vi "02 HEWH Heat Up Test SM1.vi"(0 "Equipment":T7={"COM Port"="COM3", "MW100"="MW100", "AG34970"="A-34972A", "Chamber"="WT500"}, 2 "Semiphore":T1, 5 "Degree Setting":dbl=58.0, 7 "Flow rate setting":dbl=3.0, 11 "Error In":errorcluster) -> (15 "Error Out":errorcluster)   [LabVIEW 2011]
uses:
  EquipReferences.ctl
  Heating Modes.ctl
  HEWH Tank Indicator.ctl
  PowerElements.ctl
  Use Modes.ctl
  TestedFlowratesScenarios.ctl
  GEA2/HEWH_Mode.ctl
  ValveBankPositions.ctl
  Intellifaucet/Intellfaucet Mode.ctl
  Global HEWH.vi
  <vilib>/Utility/file.llb/Write To Spreadsheet File (string).vi
  <vilib>/Analysis/NI_AALBase.lvlib
panel:
  in  "mS Between Serial Polls":u32=500
  out "Retries":i32
  out "Serial Read OK":bool
  out "GEA2":T1
  in  "Test Condition":T2=enum."Global, Tank"
  out "Chanel List":string
  out "Label Array":string[](array[string])
  out "Use Agilent?":bool
  out "Voltage":dbl=240.0
  out "T4":i32=10000
  out "COM Port":refnum<visa-resource-name>
  out "Serial Data In":string
  out "Error Serial":errorcluster
  in  "StopSerial":bool
  out "LAN IP Address":string="192.168.25.3"
  out "Computer Name":string
  in  "Mode Set?":bool
  out "Ver.":string
  out "HEATUP TEST STATUS":string
  in  "Stop":bool
  in  "Help":bool
  out "POWER":T3
  out "Tank Display":T4 {"TC6" format="%.2g"; "TIN" format="%.2g"; "TOUT" format="%.2g"; "Mean" format="%.2f"; "Std Dev" format="%.2f"; "TC5" format="%.2g"; "TC4" format="%.2g"; "TC3" format="%.2g"; "TC2" format="%.2g"; "TC1" format="%.2g"}
  in  "Function Tab":enum32{"Setup", "Test Status", "Charts"}(tab)
  out "MW100":refnum<visa-resource-name>
  out "FileName":path
  in  "Working File Directory":path=path "c:/data"
  out "T1":u32=250
  out "T2":u32=500
  out "T3":u32=500
  in  "Cold Water Available?":bool=TRUE
  out "Heating  Mode":T5=enum."Hybrid Heating"
  in  "DRM Mode":T6=3 items=["CRITICAL", "HIGH", "MEDIUM", "Normal"]
  in  "Save File Directory":path=path "c:/data"
  out "Data Array":string[][](array[string])
  out "GEA2 HyperData":bool=TRUE
  in  "Expansion Tank?":bool=TRUE
  in  "Com Err Limit":dbl=20.0
  in  "Status Tab":T8(tab)=enum."Feedback 6"
  out "errorset mode":errorcluster
  out "Init Complete":bool
  out "Mode":T9=enum."HighDemand"
  out "Set Point":u8=140
  out "Heat Source Indicator":bool
  in  "SkipStabilize":bool
  out "error stabilize":errorcluster
  out "Elapsed Time (secs)":dbl format="%.2f"
  in  "Stability Sample Delay(s)":dbl=120.0
  out "1.Delay Mins(30)":dbl
  in  "1.SkipDelay":bool
  out "Flowrate adj":dbl=3.0
  out "Error Out 1":errorcluster
  out "Downspout Flow Chart":dbl(graph)=3.8899999999999997
  out "Temp Band(+/- F)":dbl=50.0
  in  "Time Delay(30)":dbl=30.0
  out "Temp adj":dbl=3.0
  out "Downspout Temp":dbl(graph)=3.8899999999999997
  out "2.Bottom Source Indicator":bool
  out "2.TotWater":dbl
  in  "2. Initial Draw":dbl=10.75
  out "3.WaitTime(10min)":dbl
  out "error 3":errorcluster
  out "3.Heat Source Indicator":bool
  in  "Wait Time(600s)":dbl=600.0
  out "4.Delay Remaining (300s)":dbl
  in  "Delay(300s)":dbl=300.0
  in  "4.Skip Delay":bool
  out "Error 5":errorcluster
  out "Downspout Flow Chart":dbl(graph)=3.8899999999999997
  out "Downspout Flow":dbl=3.8899999999999997
  out "Total Gal Out":dbl
  out "5.Top Source Indicator":bool
  in  "Eheat Gal Limit":dbl=40.0
  in  "Flow Adjust Time (3s)":dbl=1.5
  in  "K(0.1)":dbl=0.1
  in  "Total Gal Limit":dbl=200.0
  out "6.Bottom Source Indicator":bool
  in  "Skip Waiting for Bottom Source to turn off.":bool
  out "7.Heat Source Indicator":bool
  out "Mean Tank Temp":dbl
  in  "Min Ave Temp Limit":dbl=120.0
  in  "8.Skip Waiting":bool
  out "Seconds to Completion":dbl
  in  "8.Delay(1800s)":dbl=1800.0
  out "LoggingStopped":bool=TRUE
  out "Error History":string[](array[string])
  out "Com History":string[](array[string])
  out "error datalogging":errorcluster={"status"=TRUE, "code"=-1073807346, "source"="VISA Read in Gather Test Data.vi"}
  out "St.Logging":bool
  out "Number of Records":i32
  out "Test Data":string[][](array[string])
  in  "Graph Tab":enum32{"Temperature", "Power", "Gallons"}(tab)
  out "Temps":T10(graph) caption="Waveform Chart"
  out "Ave Temp":dbl format="%0.2f"
  out "Watt Chart":T11(graph)
  out "Watts":dbl
  out "Gallons Chart":dbl(graph)
  out "Gallons":dbl
  out "Elapsed Time":dbl format="%<%H:%M:%S>t"
  in  "Stop Logging":bool
  out "Local?":bool
  # "Select the Modes for the test.  This will need to be\nset up on the water heater."
  # "Wait for stabilization.  Checks heat sources every second.  \nIf the heat sources are both off, the water heater is stabilized. \nFor StdElect. Looks at the heating element.  For other heating\nmodes, looks at the RS232 feedback on fans and compressor."
  # "\"1.\tAfter unit has been stable for 30+/-5 minutes, Open valve,\n and draw 10.75 +/- .25 gallons of water at a rate of 3+/-.25 gpm.\""
  # "First, Allow the water temp and flow to stabilize in the downspout,\nthen switch to the tank."
  # "\"2.\tIf lower heat source energizes (Hybrid Mode/eHeat Mode = FAN ON\nfollow by Compressor, Standard Electric Mode = Lower Element ON) \nbefore 10.75 gallons, then continue drawing water until Upper element \nengages as shown in step 5 (skip to step 5).\""
  # "\"3.\tIf lower heat source does not energize during 10.75 gallon draw, then wait a maximum of 10 minutes to see if lower heat source will energize.  If it does, then\nallow the water heater to recover to set point.\""
  # "\"4.\tAllow unit to sit 5 to 10 minutes in stabilized conditions, then:\""
  # "Change delay value to skip ahead."
  # "\"5.\tOpen valve and draw water at 3+/-.25 gpm until the Upper Element \nenergizes.  Water draw must stop within 5 seconds after Upper Element \nenergizes.  NOTE: when running the unit in e-Heat mode, (no upper \nelement) draw 40+/-0.25 gallons of water.\""
  # "\"6.\tIn Hybrid Mode: when the Upper Element stops and \nswitches to Lower Element, switch the unit to eHeat Mode.  \nThis will switch the lower heating source to Compressor.\""
  # "Since there may be a significant delay \nfor the compressor to turn on, also check \nto make sure that the mean tank temp\nis above some limit."
  # "7.\tAllow water heater to stabilize this second time. \n(Recover water temperature back to set point)."
  # "8.\tAllow unit to sit a minimum of 30 minutes in stabilized conditions, then;"
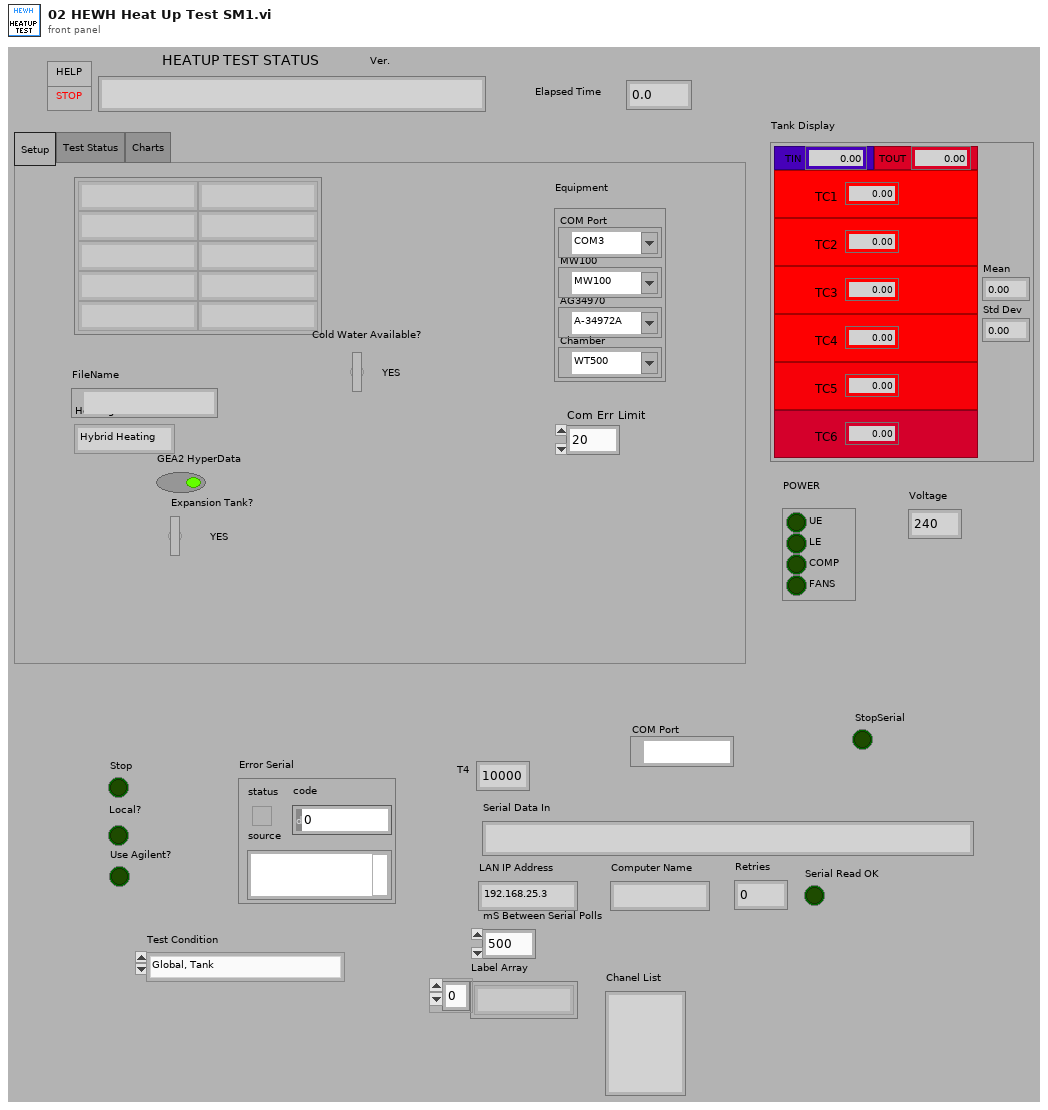
[diagram p1: front panel]
types:
  T1 = typedef "Semaphore RefNum" = refnum<k1>
  T2 = typedef "TestedFlowratesScenarios.ctl" = enum16{"DRK500,Station1", "DRK375,Lab", "SRK500,Station1,5GPM FR", "DRK375,STATION3,1/2\"HOSE", "DRK500,Station1,downspout", "DRK375,Station3,thruEcocute", "DRK375,Station3,purge", "Build2,2B,Purge", "Global, Purge", "Global, Tank"}
  T3 = typedef "PowerElements.ctl" = cluster{"UE":bool, "LE":bool, "COMP":bool, "FANS":bool}
  T4 = typedef "HEWH Tank Indicator.ctl" = cluster{"TC1-D":bool, "TC2-D":bool, "TC3-D":bool, "TC4-D":bool, "TC5-D":bool, "RTD_IN":bool, "RTDOUT":bool, "TC1":dbl, "TC2":dbl, "TC3":dbl, "TC4":dbl, "TC5":dbl, "TIN":dbl, "TOUT":dbl, "Std Dev":dbl, "Mean":dbl, "TC6-D":bool, "TC6":dbl}
  T5 = typedef "Heating Modes.ctl" = enum16{"Standard Electric", "Hybrid Heating", "E-Heat Mode"}
  T6 = typedef "Use Modes.ctl" = u16
  T7 = typedef "EquipReferences.ctl" = cluster{"COM Port":refnum<visa-resource-name>, "MW100":refnum<visa-resource-name>, "AG34970":refnum<visa-resource-name>, "Chamber":refnum<visa-resource-name>}
  T8 = enum32{"External Program Controls", "External Program Controls 2", "Program Controls", "Feedback", "Feedback 2", "Feedback 3", "Feedback 4", "Feedback 5", "Feedback 6", "Feedback 7", "Feedback 8", "Feedback 9", "Feedback 10"}
  T9 = typedef "HEWH_Mode.ctl" = enum16{"Hybrid", "StdElectric", "eHeat", "HighDemand", "Vacation"}
  T10 = cluster{"Tc Tree[0]":dbl, "Tc Tree[1]":dbl, "Tc Tree[2]":dbl, "Tc Tree[3]":dbl, "Tc Tree[4]":dbl, "Tc Tree[5]":dbl}[]
  T11 = cluster{"[0]":dbl, "[1]":dbl, "[2]":dbl, "[3]":dbl, "[4]":dbl, "[5]":dbl}[]
  T12 = typedef "Intellfaucet Mode.ctl" = enum16{"Adjust Temp", "Adjust Flow", "Start Flow", "Stop Flow"}
  T13 = typedef "ValveBankPositions.ctl" = enum16{"Heating", "Purge", "Resting", "Draw"}
  T14 = enum16{"Computation Start", "Computation stop", "Reset Computation", "Clear Computation"}
  T15 = typedef "FileVersionInformation.ctl" = cluster{"FileVersion":string, "ProductName":string, "InternalName":string, "CompanyName":string, "LegalCopyright":string, "FileDescription":string}
  T16 = enum16{"Computation Start", "Computation stop", "Reset Computation", "Clear Computation"}[]
  T17 = typedef "PowerData.ctl" = cluster{"Voltage":dbl, "Current":dbl, "Power":dbl, "WattHours":dbl}
  T18 = cluster{"Tc Tree[0]":dbl, "Tc Tree[1]":dbl, "Tc Tree[2]":dbl, "Tc Tree[3]":dbl, "Tc Tree[4]":dbl, "Tc Tree[5]":dbl}
  T19 = cluster{"[0]":dbl, "[1]":dbl, "[2]":dbl, "[3]":dbl, "[4]":dbl, "[5]":dbl}
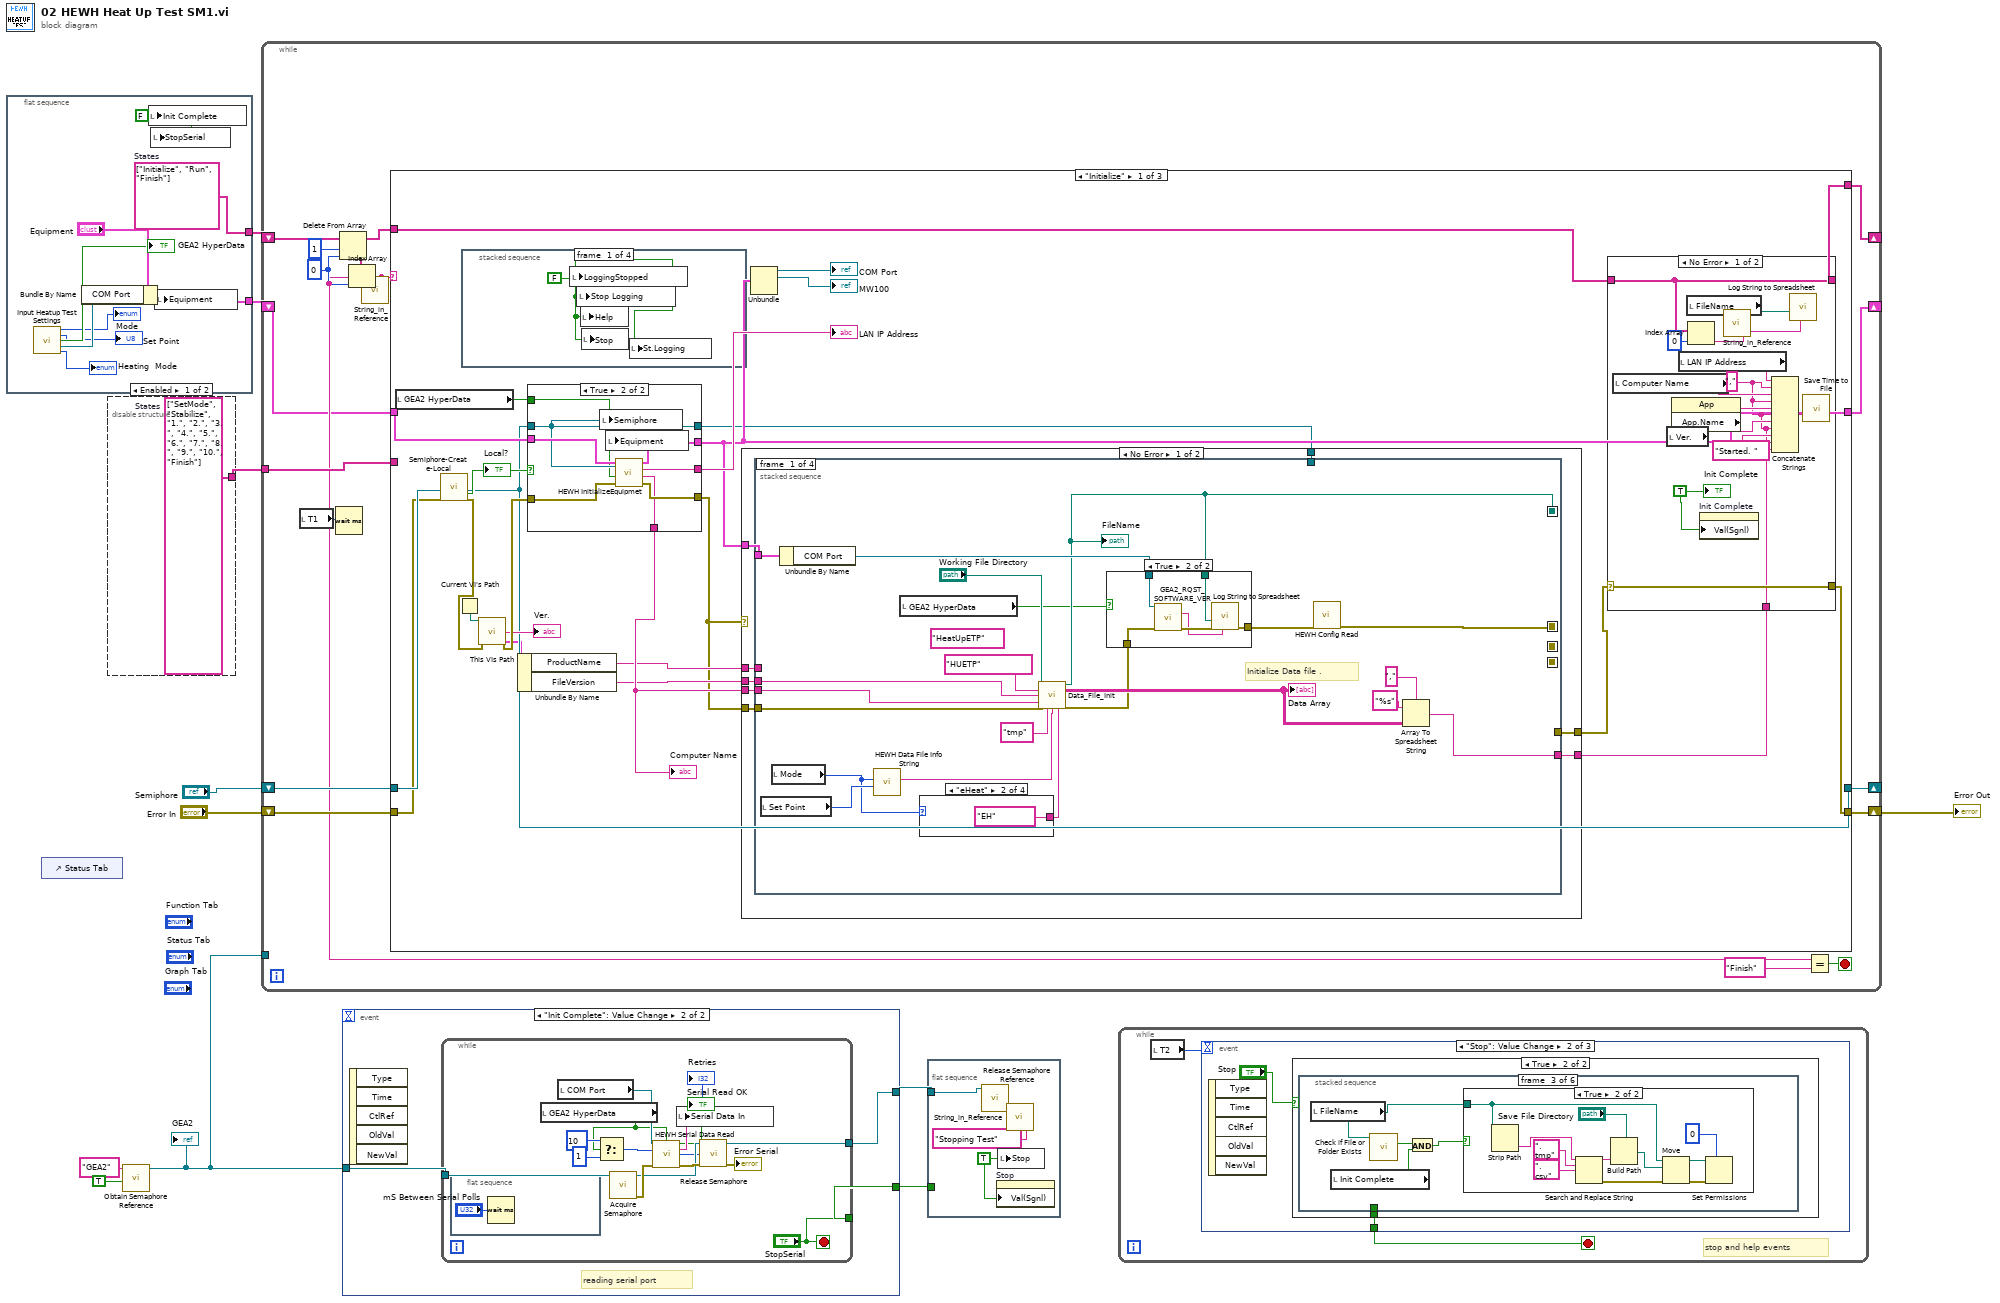
[diagram p0: block diagram]
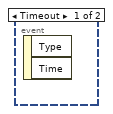
[diagram p2: hidden frame]
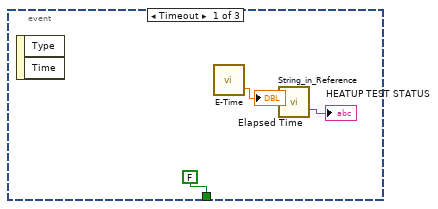
[diagram p3: hidden frame]
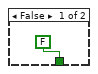
[diagram p4: hidden frame]
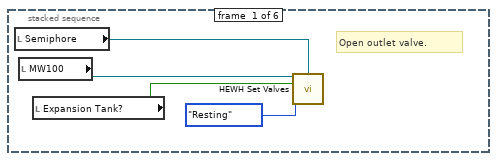
[diagram p5: hidden frame]
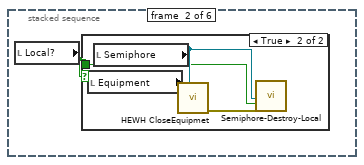
[diagram p6: hidden frame]
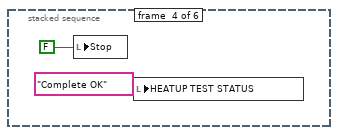
[diagram p9: hidden frame]
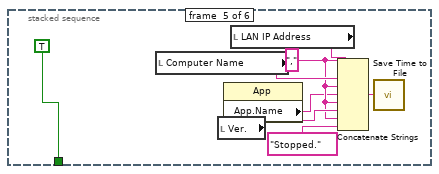
[diagram p10: hidden frame]
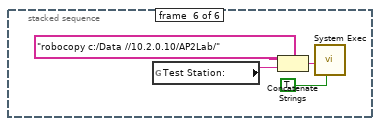
[diagram p11: hidden frame]
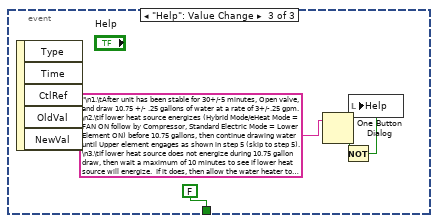
[diagram p12: hidden frame]
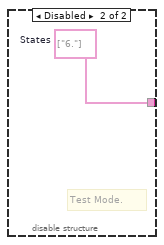
[diagram p13: hidden frame]
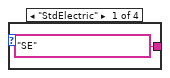
[diagram p15: hidden frame]
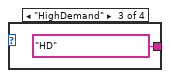
[diagram p16: hidden frame]
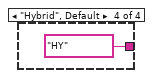
[diagram p17: hidden frame]
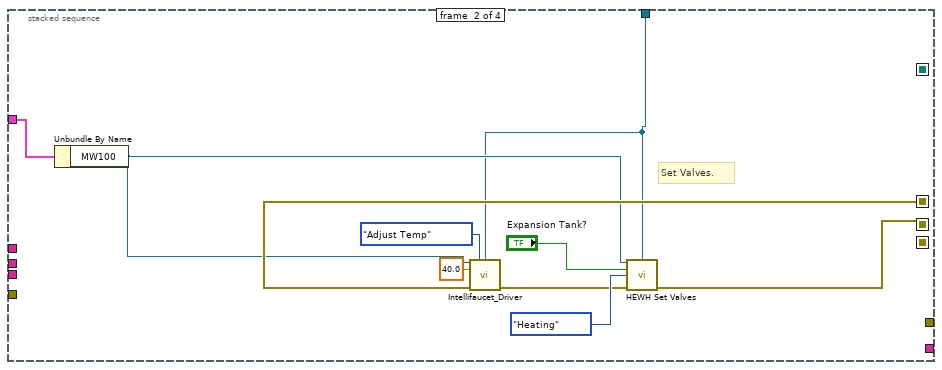
[diagram p18: hidden frame]
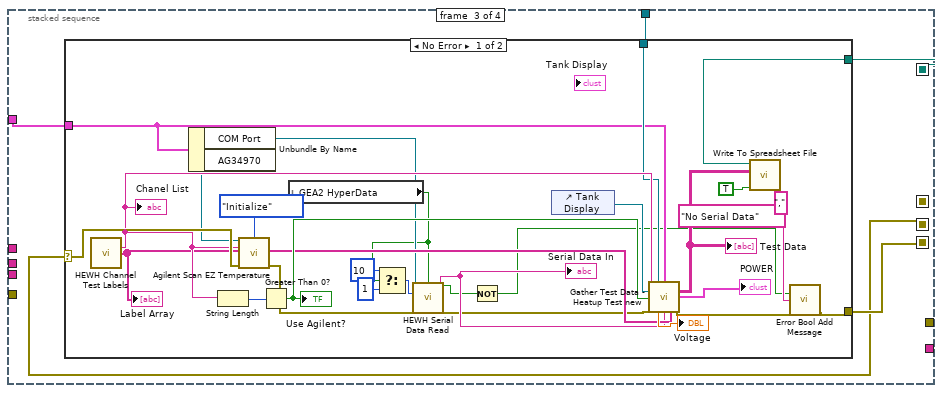
[diagram p19: hidden frame]
diagram:
  n1 = flat-sequence {
    tunnel: [w20] -> w11
    tunnel: [w16] -> w4
    frame #0 {
      w19 = FALSE ("Init Complete")
      w20 = string[] ["Initialize", "Run", "Finish"]  # States
      n2 = call "Input Heatup Test Settings.vi"() -> ("GEA2 Set Mode Out"=→"Mode":T9, "Set PointOut"=→"Set Point":u8, "GEA2 HyperData Out"=→"GEA2 HyperData":bool, "COM Port Out"=w18:refnum<visa-resource-name>, "Heating  Mode Out"=→"Heating  Mode":T5)  [unwired: 11 in]
      n3 = Bundle By Name(cluster="Equipment", "COM Port"=w18) -> (w16:T7)
      n4 = local write "Init Complete"(w19) -> ()
      n5 = local write "StopSerial"(w19) -> ()
      n6 = local write "Equipment"(w16) -> ()
    }
  }
  n7 = control-ref of="Status Tab"() -> ()  [unwired: 1 out]
  n8 = disable-structure shown="Enabled" {
    disable-tunnel: [w21 w22] -> w9
    frame Enabled {
      w21 = string[] ["SetMode", "Stabilize", "1.", "2.", "3.", "4.", "5.", "6.", "7.", "8.", "9.", "10.", "Finish"]  # States
    }
    frame Disabled {
      w22 = string[] ["6."]  # States
      # "Test Mode."
    }
  }
  n9 = call <vilib>:"Obtain Semaphore Reference.vi"("create if not found (T)"=TRUE, "name (unnamed)"="GEA2") -> ("semaphore"=w1:T1)  [unwired: 3 in, 2 out]
  "GEA2" <- w1
  n10 = while {
    shift-right: [w35] -> _
    shift-left: w11 -> [w39]
    shift-right: [w33] -> w10
    shift-left: "Error In" -> [w32]
    shift-right: [w29] -> _
    shift-left: w4 -> [w23]
    tunnel: w9 -> [w28]
    shift-right: [w26] -> _
    shift-left: "Semiphore" -> [w27]
    tunnel: w1 -> [_]
    stop <- w31 stop-if-true
    w36 = 0 ("index")
    n11 = local read "T1"() -> (w25:u32)
    n12 = Wait (ms)(milliseconds to wait=w25) -> ()  [unwired: 1 out]
    n13 = Delete From Array(array=w39, length=1, index=w36) -> (deleted portion=w37:string[], array with subset deleted=w34:string[])
    n14 = Index Array(array=w37, index=w36) -> (element=w24:string)
    n15 = call "String_in_Reference.vi"("String"=w24) -> ()  [unwired: 18 in, 1 out]
    n16 = case shown="\"Initialize\"" w24 {
      tunnel: [w61 w206 w1100] -> w35
      tunnel: w34 -> [w62 w206 w1101]
      tunnel: [w63 w204 w1102] -> w33
      tunnel: w32 -> [w58 w209 w1098]
      tunnel: w23 -> [w64 w208 w1097]
      tunnel: [w48 w208 w1097] -> w29
      tunnel: w28 -> [_ w210 _]
      tunnel: w27 -> [w59 w207 w1099]
      tunnel: [w52 w207 w1099] -> w26
      frame "Initialize" {
        n17 = local read "GEA2 HyperData"() -> (w41:bool)
        n18 = call "Semiphore-Create-Local.vi"("Semiphore"=w59, "error in (no error)"=w58) -> ("semaphore"=w52:T1, "Local?"=w60:bool, "error out"=w56:errorcluster)  [unwired: 15 in]
        "Local?" <- w60
        n19 = Current VI's Path() -> (path=w57:path)
        n20 = stacked-sequence {
          frame #0 {
            w164 = FALSE ("BottomHeater")
            n21 = local write "LoggingStopped"(w164) -> ()
            n22 = local write "Stop Logging"(w164) -> ()
            n23 = local write "Help"(w164) -> ()
            n24 = local write "Stop"(w164) -> ()
            n25 = local write "St.Logging"(w164) -> ()
          }
          frame #1 {
            n26 = Select(t=2.0, s="Cold Water Available?", f=55.0) -> (s? t:f=→"Temp Band(+/- F)":dbl)
          }
          frame #2 {
            # "Data Log Sample Rate"
            # "Loop Delay"
            # "Decision Sampling"
            # "Control Loop Rate"
            "T1" <- u32 250
            "T2" <- u32 500 ("T2")
            "T3" <- u32 500 ("T3")
            "T4" <- 10000 ("T4")
          }
          frame #3 {
            w173 = errorcluster {"status"=FALSE, "code"=0, "source"=""} ("Error Out")
            n27 = local write "Error Out 1"(w173) -> ()
            n28 = local write "Error Out"(w173) -> ()
            n29 = local write "Error 5"(w173) -> ()
            n30 = local write "error 3"(w173) -> ()
          }
        }
        n31 = call "This VIs Path.vi"("path"=w57, "error in (no error)"=w56) -> ("File Version Info"=→"Ver.":string, "FileVersionInfo Out"=w44:T15, "error out"=w55:errorcluster)  [unwired: 9 in, 2 out]
        n32 = Unbundle By Name(w44) -> ("ProductName"=w43:string, "FileVersion"=w42:string)
        n33 = case shown="True" w60 {
          tunnel: w55 -> [w195 w203]
          tunnel: w64 -> [w194 w200]
          tunnel: [w194 w201] -> w48
          tunnel: [w195 w202] -> w40
          tunnel: w52 -> [w191 w197]
          tunnel: [w193 w199] -> w46
          tunnel: [w192 w198] -> w51
          tunnel: [w191 w197] -> w47
          tunnel: w41 -> [_ w196]
          frame False {
            n34 = call "IP and Computer Name.vi"() -> ("IP Address"=w192:string, "Computer Name"=w193:string)  [unwired: 10 in]
          }
          frame True {
            n35 = local write "Semiphore"(w197) -> ()
            n36 = call "HEWH InitializeEquipmet.vi"("Semiphore"=w197, "Error In"=w203, "GEA2?"=w196, "Equipment"=w200) -> ("Error Out"=w202:errorcluster, "Computer Name"=w199:string, "LAN IP Address"=w198:string, "Equipment Out"=w201:T7)  [unwired: 4 in]
            n37 = local write "Equipment"(w201) -> ()
          }
        }
        "Computer Name" <- w46
        "LAN IP Address" <- w51
        n38 = case shown="No Error" w40 {
          tunnel: [w72 w163] -> w49
          tunnel: w40 -> [w71 w163]
          tunnel: w48 -> [w70 _]
          tunnel: w47 -> [w69 _]
          tunnel: w46 -> [w68 _]
          tunnel: [w67 "Error Init." ("spreadsheet string")] -> w45
          tunnel: w43 -> [w66 _]
          tunnel: w42 -> [w65 _]
          frame No Error {
            n39 = stacked-sequence {
              seq-local: [_ w114 _ _] -> [_ _ w115 _]
              seq-local: [w82 _ _ _] -> [_ w109 _ _]
              seq-local: [_ _ w117 _] -> [_ _ _ w154]
              seq-local: [w77 _ _ _] -> [_ _ w116 _]
              tunnel: [_ _ _ w155] -> w72
              tunnel: w68 -> [w93 _ _ _]
              tunnel: w71 -> [w92 _ _ _]
              tunnel: w70 -> [w79 w113 w119 _]
              tunnel: w69 -> [_ w105 w118 w152]
              tunnel: [w85 _ _ _] -> w67
              tunnel: w66 -> [_ _ _ _]
              tunnel: w65 -> [w89 _ _ _]
              frame #0 {
                (unwired) "HeatUpETP" ("Test_Type In:")
                # "Initialize Data file ."
                n40 = local read "Set Point"() -> (w84:u8)
                n41 = local read "Mode"() -> (w76:T9)
                n42 = Unbundle By Name(w79) -> ("COM Port"=w78:refnum<visa-resource-name>)
                n43 = call "HEWH Data File Info String.vi"("Set PointOut"=w84, "GEA2 Set Mode"=w76) -> ("Info string"=w83:string)  [unwired: 9 in]
                n44 = local read "GEA2 HyperData"() -> (w73:bool)
                n45 = case shown="\"eHeat\"" w76 {
                  tunnel: ["SE" ("Mode:") "EH" ("Mode:") "HD" ("Mode:") "HY" ("Mode:")] -> w75
                  frame "StdElectric" {
                  }
                  frame "eHeat" {
                  }
                  frame "HighDemand" {
                  }
                  frame "Hybrid", Default {
                  }
                }
                n46 = call "Data_File_Init.vi"("Data File Directory"="Working File Directory", "Test_Name In:"="HUETP", "Version In:"=w89, "Computer Name In:"=w93, "error in (no error)"=w92, "File Extension:"="tmp", "Ambient Temp / RH:"=w83, "Mode:"=w75) -> ("FileName"=w77:path, "Data Array"=w86:string[][], "error out"=w81:errorcluster)  [unwired: 5 in]
                "FileName" <- w77
                "Data Array" <- w86
                n47 = case shown="True" w73 {
                  tunnel: w81 -> [w94 w100]
                  tunnel: [w94 w98] -> w80
                  tunnel: w78 -> [_ w97]
                  tunnel: w77 -> [_ w95]
                  frame False {
                  }
                  frame True {
                    n48 = call "GEA2_RQST_SOFTWARE_VER.vi"("ComPort"=w97, "Error In"=w100) -> ("Software Version"=w96:string, "Error Out"=w99:errorcluster)  [unwired: 10 in, 2 out]
                    n49 = call "Log String to Spreadsheet.vi"("String"=w96, "error in (no error)"=w99, "FileName"=w95) -> ("error out"=w98:errorcluster)  [unwired: 8 in]
                  }
                }
                n50 = call "HEWH Config Read.vi"("error in (no error)"=w80) -> ("error out"=w82:errorcluster)  [unwired: 13 in, 1 out]
                n51 = Array To Spreadsheet String(delimiter (Tab)=",", array=w86, 3:"%s" ("format string")) -> (spreadsheet string=w85:string)
              }
              frame #1 {
                # "Set Valves."
                n52 = Unbundle By Name(w113) -> ("MW100"=w108:refnum<visa-resource-name>)
                n53 = call "Intellifaucet_Driver.vi"("VISA session"=w108, "Mode"=Intellfaucet_Mode."Adjust Temp", "Semiphore"=w105, "Temperature(F)"=40.0, "Error In"=w109) -> ("Error Out"=w110:errorcluster)  [unwired: 9 in, 1 out]
                n54 = call "HEWH Set Valves.vi"("VISA session"=w108, "Semiphore"=w105, "Expansion Tank?"="Expansion Tank?", "Valve Bank Setting"=ValveBankPositions."Heating", "Error In"=w110) -> ("Error Out"=w114:errorcluster)  [unwired: 9 in, 1 out]
              }
              frame #2 {
                n55 = case shown="No Error" w115 {
                  selector: w115 -> [w148 w149]
                  tunnel: w119 -> [w139 _]
                  tunnel: w118 -> [w143 _]
                  tunnel: [w124 w149] -> w117
                  tunnel: w116 -> [w134 _]
                  frame No Error {
                    n56 = call "HEWH Channel Test Labels.vi"() -> ("Chanel List"=w144:string, "Label List"=w141:string[])  [unwired: 13 in, 1 out]
                    "Chanel List" <- w144
                    "Label Array" <- w141
                    n57 = Unbundle By Name(w139) -> ("COM Port"=w138:refnum<visa-resource-name>, "AG34970"=w137:refnum<visa-resource-name>)
                    n58 = String Length(string=w144) -> (length=w146:i32)
                    n59 = call "Agilent Scan EZ Temperature.vi"("VISA Resource Name"=w137, "Control"=enum16{"Initialize", "Read", "Experiment"}."Initialize", "Channel Input"=w144, "error in (no error)"=w148) -> ("error out"=w140:errorcluster)  [unwired: 8 in, 3 out]
                    n60 = Greater Than 0?(x=w146) -> (x > 0?=w145:bool)
                    "Use Agilent?" <- w145
                    n61 = local read "GEA2 HyperData"() -> (w127:bool)
                    n62 = Select(t=10, s=w127, f=1) -> (s? t:f=w126:i32)
                    n63 = call "HEWH Serial Data Read.vi"("Serial Port Ref"=w138, "GEA2 HyperData"=w127, "Retries"=w126, "error in (no error)"=w140) -> ("Serial Read OK"=w125:bool, "Read String"=w133:string, "error out"=w120:errorcluster)  [unwired: 8 in, 1 out]
                    "Serial Data In" <- w133
                    n64 = Not(x=w125) -> (.not. x?=w121:bool)
                    n65 = control-ref of="Tank Display"() -> (w132:refnum<vi>)
                    n66 = call "Gather Test Data - Heatup Test new.vi"("Agilent Scan List"=w144, "Semiphore"=w143, "Equipment"=w139, "Tank Display Ref"=w132, "Agilent?"=w145, "error in (no error)"=w120, "Serial Data In"=w133, "Agilent Label Array"=w141) -> ("Output Data"=w131:string[][], "POWER"=→"POWER":T3, "Voltage"=→"Voltage":dbl, "error out"=w123:errorcluster)  [unwired: 2 in, 2 out]
                    "Test Data" <- w131
                    n67 = call-poly <vilib>:"Write To Spreadsheet File.vi"("delimiter (\\t)"="," ("delimiter (\\t)"), "append to file? (new file:F)"=TRUE, "2D data"=w131, "file path (dialog if empty)"=w134) -> ()  [unwired: 4 in, 1 out]
                    n68 = call "Error Bool Add Message.vi"("Error?"=w121, "Message"="No Serial Data", "Error In"=w123) -> ("Error Out"=w124:errorcluster)  [unwired: 12 in]
                  }
                  frame Error {
                  }
                }
              }
              frame #3 {
                w156 = T16 [enum."Computation Start", enum."Reset Computation"] items=["Computation Start", "Computation stop", "Reset Computation", "Clear Computation"]
                # "Reset and restart computation of gallons."
                n69 = local read "MW100"() -> (w150:refnum<visa-resource-name>)
                n70 = call "HEWH Totalize Flow Control.vi"("VISA session"=w150, "Semiphore"=w152, "Totalize Flow"=FALSE, "error in (no error)"=w154) -> ("error out"=w153:errorcluster)  [unwired: 10 in, 1 out]
                n71 = for {
                  tunnel: w156 -> [w159] mode=indexing
                  shift-right: [w160] -> w155
                  shift-left: w153 -> [w161]
                  tunnel: w152 -> [w158]
                  tunnel: w150 -> [w157]
                  n72 = call "YKMW100 Computation Control.vi"("VISA session"=w157, "Semiphore"=w158, "Mode"=w159, "error in (no error)"=w161) -> ("error out"=w160:errorcluster)  [unwired: 10 in, 1 out]
                }
              }
            }
          }
          frame Error {
          }
        }
        n73 = Unbundle(w48) -> ("COM Port"=→"COM Port":refnum<visa-resource-name>, "MW100"=→"MW100":refnum<visa-resource-name>)  [unwired: 2 out]
        n74 = case shown="No Error" w49 {
          selector: w49 -> [w188 w190]
          tunnel: [w183 string[] ["Finish"] ("States")] -> w61
          tunnel: w62 -> [w183 _]
          tunnel: [w188 w190] -> w63
          tunnel: w45 -> [w174 _]
          frame No Error {
            w175 = ","
            w182 = TRUE ("Init Complete")
            n75 = local read "Computer Name"() -> (w176:string)
            n76 = local read "Ver."() -> (w177:string)
            n77 = property class="App"() -> ("App.Name"=w179:string)  [unwired: 2 in, 2 out]
            n78 = local read "LAN IP Address"() -> (w180:string)
            n79 = local read "FileName"() -> (w185:path)
            n80 = Index Array(array=w183, index=0) -> (element=w186:string)
            n81 = property on="Init Complete" class="Bool (strict)"("Val(Sgnl)"=w182) -> ()  [unwired: 2 in, 2 out]
            n82 = call "String_in_Reference.vi"("String"=w186) -> ("String Out"=w184:string)  [unwired: 18 in]
            n83 = Concatenate Strings(w180, w175, w176, w175, w179, w175, w177, w175, "Started. " ("string"), w175, w174) -> (w181:string)
            n84 = call "Log String to Spreadsheet.vi"("String"=w184, "FileName"=w185) -> ()  [unwired: 9 in, 1 out]
            n85 = call "Save Time to File.vi"("String"=w181) -> ()  [unwired: 13 in, 2 out]
            "Init Complete" <- w182
          }
          frame Error {
            n86 = call <vilib>:"Simple Error Handler.vi"("error in (no error)"=w190) -> ()  [unwired: 4 in, 5 out]
          }
        }
      }
      frame "Run" {
        n87 = while {
          shift-right: [w226] -> _
          shift-left: w210 -> [w227]
          tunnel: w208 -> [w223]
          tunnel: w207 -> [w222]
          shift-right: [w212] -> w204
          shift-left: w209 -> [w221]
          stop <- w217 stop-if-true
          w228 = 0 ("index")
          # "Error State shows both upper and lower elements on."
          # "Water Draw Test Sequence"
          n88 = local read "Stop Logging"() -> (w214:bool)
          n89 = local read "Heating  Mode"() -> (w211:T5)
          n90 = flat-sequence {
            tunnel: w221 -> [w235]
            tunnel: [w235] -> w220
            tunnel: [w231] -> w218
            tunnel: w213 -> [w231]
            frame #0 {
              n91 = local read "FileName"() -> (w233:path)
              n92 = control-ref of="Status Tab"() -> (w234:refnum<vi>)
              n93 = call "String_in_Reference.vi"("String"=w231) -> ("String Out"=w232:string)  [unwired: 18 in]
              n94 = call "Tab Control - Change to TabName Heatup.vi"("Label.Text"=w231, "Tab Control Heatup"=w234) -> ()  [unwired: 9 in]
              n95 = call "Log String to Spreadsheet.vi"("String"=w232, "FileName"=w233) -> ()  [unwired: 9 in, 1 out]
            }
          }
          n96 = Delete From Array(array=w227, length=1, index=w228) -> (deleted portion=w229:string[], array with subset deleted=w225:string[])
          n97 = Index Array(array=w229, index=w228) -> (element=w216:string)
          n98 = local read "T1"() -> (w219:u32)
          n99 = Wait (ms)(milliseconds to wait=w219) -> ()  [unwired: 1 out]
          n100 = Select(t="Finish", s=w214, f=w216) -> (s? t:f=w213:string)
          n101 = case shown="\"Stabilize\"" w213 {
            tunnel: w220 -> [w239 w289 w362 w459 w535 w631 w721 w750 w839 w932 w975 w992 w998]
            tunnel: [w236 w294 w366 w472 w543 w638 w723 w761 w841 w930 w974 w991 w994] -> w212
            tunnel: [w241 w293 w365 w471 w542 w637 w724 w762 w842 w929 w972 w993 w1002] -> w226
            tunnel: w225 -> [w240 w292 w364 w470 w537 w636 w724 w763 w836 w929 w972 w993 w1002]
            tunnel: w223 -> [_ _ _ w469 _ _ _ _ _ _ _ _ _]
            tunnel: w222 -> [w237 w290 w360 w466 w536 w630 w719 w748 w840 w931 _ _ w997]
            tunnel: w211 -> [_ _ _ _ _ _ _ w764 w837 _ _ _ _]
            frame "SetMode" {
              n102 = while {
                tunnel: w239 -> [w245]
                tunnel: [w244] -> w238
                tunnel: w237 -> [w243]
                stop <- w246 stop-if-true
                # "Remove Double\nchecking mode \nset."
                n103 = disable-structure shown="Enabled" {
                  disable-tunnel: [w249 TRUE ("T button?")] -> w247
                  disable-tunnel: "DRM Mode" -> [w248 _]
                  frame Disabled {
                    n104 = call "Mode.vi"("Mode"=w248) -> ("T button?"=w249:bool)  [unwired: 10 in]
                  }
                  frame Enabled {
                  }
                }
                n105 = case shown="True" w247 {
                  tunnel: [FALSE TRUE] -> w246
                  tunnel: w245 -> [w251 w259]
                  tunnel: [w251 w258] -> w244
                  tunnel: w243 -> [_ w261]
                  tunnel: "DRM Mode" -> [_ w262]
                  frame False {
                    n106 = while {
                      stop <- "Mode Set?" stop-if-true
                      w253 = TRUE ("Visible")
                      # "wait for correct \nmode setting"
                      n107 = property on="Mode Set?" class="Bool"("Blinking"=w253) -> ()  [unwired: 2 in, 2 out]
                      n108 = property on="Mode Set?" class="Bool"("Visible"=w253) -> ()  [unwired: 2 in, 2 out]
                      n109 = Wait (ms)(milliseconds to wait=u32 250) -> ()  [unwired: 1 out]
                    }
                  }
                  frame True {
                    w264 = FALSE ("Visible")
                    # "set mode of drm"
                    n110 = local read "MW100"() -> (w257:refnum<visa-resource-name>)
                    n111 = local read "GEA2 HyperData"() -> (w256:bool)
                    n112 = call "HEWH Set DRM Mode.vi"("MW100"=w257, "Semiphore"=w261, "Mode"=w262, "error in (no error)"=w259) -> ("error out"=w260:errorcluster)  [unwired: 11 in]
                    n113 = case shown="True" w256 {
                      tunnel: w260 -> [w265 w271]
                      tunnel: [w265 w266] -> w258
                      frame False {
                      }
                      frame True {
                        n114 = local read "GEA2"() -> (w267:T1)
                        n115 = call <vilib>:"Acquire Semaphore.vi"("error in (no error)"=w271, "semaphore"=w267) -> ("error out"=w270:errorcluster, "semaphore out"=w268:T1)  [unwired: 3 in, 1 out]
                        n116 = local read "COM Port"() -> (w272:refnum<visa-resource-name>)
                        n117 = local read "Set Point"() -> (w273:u8)
                        n118 = local read "Mode"() -> (w274:T9)
                        n119 = call "HEWH GEA2 Set Tank Mode and Temp.vi"("ComPort"=w272, "Mode"=w274, "Set Point"=w273, "Error In"=w270) -> ("Error Out"=w269:errorcluster)  [unwired: 9 in, 2 out]
                        n120 = call <vilib>:"Release Semaphore.vi"("error in (no error)"=w269, "semaphore"=w268) -> ("error out"=w266:errorcluster)  [unwired: 4 in, 1 out]
                      }
                    }
                    n121 = property on="Mode Set?" class="Bool"("Blinking"=w264) -> ()  [unwired: 2 in, 2 out]
                    n122 = property on="Mode Set?" class="Bool"("Visible"=w264) -> ()  [unwired: 2 in, 2 out]
                  }
                }
              }
              n123 = case shown="Error" w238 {
                selector: w238 -> [w275 w277]
                tunnel: [w276 string[] ["Finish"] ("States")] -> w241
                tunnel: w240 -> [w276 _]
                tunnel: [w275 w277] -> w236
                frame No Error {
                }
                frame Error {
                  n124 = Unbundle By Name(w277) -> ("source"=w282:string)
                  n125 = local read "FileName"() -> (w279:path)
                  n126 = Concatenate Strings("Error: " ("string"), w282) -> (w280:string)
                  n127 = call "String_in_Reference.vi"("String"=w280) -> ("String Out"=w278:string)  [unwired: 18 in]
                  n128 = call "Log String to Spreadsheet.vi"("String"=w278, "FileName"=w279) -> ()  [unwired: 9 in, 1 out]
                }
              }
              "errorset mode" <- w236
            }
            frame "Stabilize" {
              n129 = call "E-Time.vi"("error in (no error)"=w289) -> ("error out"=w287:errorcluster, "Elapsed Time (sec)"=w286:dbl)  [unwired: 8 in, 1 out]
              n130 = while {
                tunnel: w287 -> [w311]
                tunnel: [w328] -> w291
                tunnel: w290 -> [w320]
                shift-right: [w301] -> _
                shift-left: w286 -> [w304]
                tunnel: ["SkipStabilize"] -> w288
                shift-right: [w298] -> _
                shift-left: _ -> [w297]
                tunnel: [w296] -> w285
                tunnel: [w295] -> w284
                i -> [w316]
                stop <- w315 stop-if-true
                n131 = flat-sequence {
                  tunnel: [w331] -> w312
                  tunnel: w311 -> [w331]
                  frame #0 {
                    n132 = local read "T2"() -> (w332:u32)
                    n133 = Wait (ms)(milliseconds to wait=w332) -> ()  [unwired: 1 out]
                  }
                }
                n134 = local read "Use Agilent?"() -> (w307:bool)
                n135 = local read "Chanel List"() -> (w323:string)
                n136 = local read "Equipment"() -> (w324:T7)
                n137 = local read "Serial Data In"() -> (w309:string)
                n138 = local read "Label Array"() -> (w308:string[])
                n139 = control-ref of="Tank Display"() -> (w322:refnum<vi>)
                n140 = call "Gather Test Data - Heatup Test new.vi"("Agilent Scan List"=w323, "Semiphore"=w320, "Equipment"=w324, "Tank Display Ref"=w322, "Agilent?"=w307, "error in (no error)"=w312, "Serial Data In"=w309, "Agilent Label Array"=w308) -> ("Output Data"=w318:string[][], "POWER"=w321:T3, "Voltage"=w306:dbl, "error out"=w319:errorcluster)  [unwired: 2 in, 2 out]
                n141 = Equal To 0?(x=w316) -> (x = 0?=w296:bool)
                n142 = local read "St.Logging"() -> (w310:bool)
                n143 = local write "Voltage"(w306) -> ()
                n144 = local write "Test Data"(w318) -> ()
                n145 = local write "POWER"(w321) -> ()
                n146 = Unbundle(w321) -> ("UE"=w325:bool, "LE"=w326:bool, "COMP"=w327:bool, "FANS"=w314:bool)
                n147 = Compound Arithmetic op=AND(invert w325, invert w326, invert w327, invert w314) -> (w295:bool)
                n148 = Not(x=w295) -> (.not. x?=w303:bool)
                "Heat Source Indicator" <- w303
                n149 = And(x=w297, y=w295) -> (x .and. y?=w313:bool)
                n150 = Compound Arithmetic op=OR(w313, "SkipStabilize", w310) -> (w315:bool)
                n151 = Compound Arithmetic op=OR(w296, w315) -> (w317:bool)
                n152 = case shown="True" w317 {
                  tunnel: w318 -> [_ w334]
                  frame False {
                  }
                  frame True {
                    n153 = local read "FileName"() -> (w337:path)
                    n154 = Index Array(array=w334, index (row)=1) -> (element=w333:string[])  [unwired: 1 in]
                    n155 = call-poly <vilib>:"Write To Spreadsheet File.vi"("delimiter (\\t)"="," ("delimiter (\\t)"), "append to file? (new file:F)"=TRUE, "1D data"=w333, "file path (dialog if empty)"=w337) -> ()  [unwired: 4 in, 1 out]
                  }
                }
                n156 = call "E-Time.vi"("error in (no error)"=w319) -> ("error out"=w328:errorcluster, "Elapsed Time (sec)"=w302:dbl)  [unwired: 8 in, 1 out]
                "Elapsed Time (secs)" <- w302
                n157 = case shown="True" w303 {
                  tunnel: [w329 w330] -> w301
                  tunnel: w302 -> [_ w330]
                  tunnel: w304 -> [w329 _]
                  frame False {
                  }
                  frame True {
                  }
                }
                n158 = Subtract(x=w302, y=w301) -> (x-y=w300:dbl)
                n159 = Greater Or Equal?(x=w300, y="Stability Sample Delay(s)") -> (x >= y?=w298:bool)
              }
              n160 = case shown="No Error" w291 {
                selector: w291 -> [w345 w353]
                tunnel: [w343 string[] ["Finish"] ("States")] -> w293
                tunnel: w292 -> [w342 _]
                tunnel: [w345 w353] -> w294
                tunnel: w288 -> [w344 _]
                tunnel: w285 -> [w340 _]
                tunnel: w284 -> [w339 _]
                frame No Error {
                  n161 = And(x=w339, y=w340) -> (x .and. y?=w341:bool)
                  n162 = case shown="True" w344 {
                    frame False {
                    }
                    frame True {
                      n163 = local read "FileName"() -> (w352:path)
                      n164 = call "String_in_Reference.vi"("String"="Skip Stabilize " ("string")) -> ("String Out"=w351:string)  [unwired: 18 in]
                      n165 = call "Log String to Spreadsheet.vi"("String"=w351, "FileName"=w352) -> ()  [unwired: 9 in, 1 out]
                    }
                  }
                  n166 = case shown="True" w341 {
                    tunnel: [w346 w349] -> w343
                    tunnel: w342 -> [w346 w348]
                    frame False {
                    }
                    frame True {
                      n167 = Build Array (concatenate)("Predraw " ("string"), w348) -> (w349:string[])
                    }
                  }
                }
                frame Error {
                  n168 = Unbundle By Name(w353) -> ("source"=w358:string)
                  n169 = local read "FileName"() -> (w355:path)
                  n170 = Concatenate Strings("Error: " ("string"), w358) -> (w356:string)
                  n171 = call "String_in_Reference.vi"("String"=w356) -> ("String Out"=w354:string)  [unwired: 18 in]
                  n172 = call "Log String to Spreadsheet.vi"("String"=w354, "FileName"=w355) -> ()  [unwired: 9 in, 1 out]
                  "error stabilize" <- w353
                }
              }
            }
            frame "Predraw" {
              n173 = stacked-sequence {
                tunnel: w362 -> [w370 w377 w383]
                tunnel: [w369 _ _] -> _
                tunnel: w360 -> [w367 w373 w382]
                tunnel: [_ w372 _] -> _
                tunnel: [_ _ w384] -> w361
                frame #0 {
                  n174 = local read "MW100"() -> (w368:refnum<visa-resource-name>)
                  n175 = call "HEWH Totalize Flow Control.vi"("VISA session"=w368, "Semiphore"=w367, "Totalize Flow"=FALSE, "error in (no error)"=w370) -> ("error out"=w369:errorcluster)  [unwired: 10 in, 1 out]
                }
                frame #1 {
                  n176 = local read "Flow rate setting"() -> (w376:dbl)
                  n177 = local read "Degree Setting"() -> (w375:dbl)
                  n178 = local read "Temp Band(+/- F)"() -> (w378:dbl)
                  n179 = local read "Equipment"() -> (w374:T7)
                  n180 = call "Purge Water Sequence SM.vi"("Degree Setting"=w375, "Equipment"=w374, "Semiphore"=w373, "Flow rate setting"=w376, "Temp Band(+/- F)"=w378, "Error In"=w377) -> ("Error Out"=w372:errorcluster)  [unwired: 4 in, 5 out]
                }
                frame #2 {
                  n181 = local read "Expansion Tank?"() -> (w380:bool)
                  n182 = local read "MW100"() -> (w381:refnum<visa-resource-name>)
                  n183 = call "HEWH Set Valves.vi"("VISA session"=w381, "Semiphore"=w382, "Expansion Tank?"=w380, "Valve Bank Setting"=ValveBankPositions."Draw", "Error In"=w383) -> ("Error Out"=w384:errorcluster)  [unwired: 9 in, 1 out]
                }
              }
              n184 = while {
                tunnel: [w385] -> _
                tunnel: w360 -> [w417]
                shift-right: [w418] -> w363
                shift-left: w361 -> [w430]
                i -> [w423]
                stop <- w421 stop-if-true
                n185 = local read "Flow Adjust Time (3s)"() -> (w396:dbl)
                n186 = local read "T2"() -> (w428:u32)
                n187 = local read "Flow rate setting"() -> (w403:dbl)
                n188 = local read "Degree Setting"() -> (w402:dbl)
                n189 = local read "Serial Data In"() -> (w392:string)
                n190 = local read "Use Agilent?"() -> (w393:bool)
                n191 = local read "Label Array"() -> (w391:string[])
                n192 = local read "Equipment"() -> (w427:T7)
                n193 = local read "Chanel List"() -> (w426:string)
                n194 = local read "K(0.1)"() -> (w395:dbl)
                n195 = control-ref of="Tank Display"() -> (w425:refnum<vi>)
                n196 = Wait (ms)(milliseconds to wait=w428) -> ()  [unwired: 1 out]
                n197 = call "Gather Test Data - Heatup Test new.vi"("Agilent Scan List"=w426, "Semiphore"=w417, "Equipment"=w427, "Tank Display Ref"=w425, "Agilent?"=w393, "error in (no error)"=w430, "Serial Data In"=w392, "Agilent Label Array"=w391) -> ("Output Data"=w406:string[][], "POWER"=w431:T3, "Voltage"=w394:dbl, "error out"=w414:errorcluster)  [unwired: 2 in, 2 out]
                n198 = local write "POWER"(w431) -> ()
                n199 = local read "Flowrate adj"() -> (w399:dbl)
                n200 = local read "Temp adj"() -> (w398:dbl)
                n201 = local write "Voltage"(w394) -> ()
                n202 = call "E-Time.vi"("error in (no error)"=w414) -> ("error out"=w413:errorcluster, "Elapsed Time (sec)"=w412:dbl)  [unwired: 8 in, 1 out]
                n203 = local write "Test Data"(w406) -> ()
                n204 = for {
                  tunnel: string[] ["GALLONS", "FLOW(GPM)", "Tc_down"] -> [w434] mode=indexing
                  tunnel: [w433] -> w408 mode=indexing
                  tunnel: w406 -> [w432]
                  n205 = call "Array_Search_For_Num.vi"("N Rows of Data"=w432, "Title?"=w434) -> ("number"=w433:dbl)  [unwired: 12 in, 1 out]
                }
                n206 = Unbundle(w431) -> ("UE"=w387:bool, "LE"=w386:bool, "COMP"=w390:bool, "FANS"=w420:bool)
                n207 = local read "Test Condition"() -> (w415:T2)
                n208 = Index Array(array=w408, index #1=0 ("index"), index #2=1 ("index"), index #3=2 ("index")) -> (element #2=w405:dbl, element #3=w404:dbl)  [unwired: 1 out]
                n209 = local read "MW100"() -> (w416:refnum<visa-resource-name>)
                n210 = call "HEWH Flow Adjustment.vi"("VISA session"=w416, "Configuration"=w415, "Semiphore"=w417, "GPM Target(3)"=w403, "GPM reading"=w405, "Flow rate setting In"=w399, "Error In"=w413, "Elapsed Time (sec)"=w412, "Flow Adjust Time (3s)"=w396, "K(0.1)"=w395) -> ("Flow rate setting Out"=w400:dbl, "Error Out"=w419:errorcluster)  [unwired: 3 in, 1 out]
                n211 = Compound Arithmetic op=AND(w387, w386) -> (w388:bool)
                n212 = Compound Arithmetic op=OR(w386, w390, w420) -> (w389:bool)
                n213 = local read "Stop Logging"() -> (w397:bool)
                n214 = call "HEWH Temp Adjustment.vi"("VISA session"=w416, "Semiphore"=w417, "Degrees Target(58)"=w402, "Degrees reading"=w404, "Degrees setting In"=w398, "Error In"=w419, "Elapsed Time (sec)"=w412, "Temp Adjust Time (3s)"=w396, "K(0.1)"=w395) -> ("Degree setting Out"=w401:dbl, "Error Out"=w418:errorcluster)  [unwired: 4 in, 1 out]
                n215 = Compound Arithmetic op=AND(invert w388, w389) -> (w385:bool)
                n216 = local write "2.Bottom Source Indicator"(w385) -> ()
                n217 = Unbundle By Name(w418) -> ("status"=w429:bool)
                n218 = Equal To 0?(x=w423) -> (x = 0?=w422:bool)
                n219 = local write "Flowrate adj"(w400) -> ()
                n220 = local write "Temp adj"(w401) -> ()
                n221 = Compound Arithmetic op=OR(w429, w385, w397) -> (w421:bool)
                n222 = Compound Arithmetic op=OR(w422, w421) -> (w424:bool)
                n223 = case shown="True" w424 {
                  tunnel: w406 -> [_ w435]
                  frame False {
                  }
                  frame True {
                    n224 = local read "FileName"() -> (w440:path)
                    n225 = Index Array(array=w435, index (row)=1) -> (element=w438:string[])  [unwired: 1 in]
                    n226 = call-poly <vilib>:"Write To Spreadsheet File.vi"("delimiter (\\t)"="," ("delimiter (\\t)"), "append to file? (new file:F)"=TRUE, "1D data"=w438, "file path (dialog if empty)"=w440) -> ()  [unwired: 4 in, 1 out]
                  }
                }
              }
              n227 = case shown="No Error" w363 {
                selector: w363 -> [w446 w450]
                tunnel: [w447 string[] ["Finish"] ("States")] -> w365
                tunnel: w364 -> [w448 _]
                tunnel: [w445 w450] -> w366
                tunnel: w360 -> [w443 _]
                frame No Error {
                  n228 = local read "Expansion Tank?"() -> (w442:bool)
                  n229 = local read "MW100"() -> (w444:refnum<visa-resource-name>)
                  n230 = Build Array (concatenate)("Stabilize " ("string"), w448) -> (w447:string[])
                  n231 = call "HEWH Set Valves.vi"("VISA session"=w444, "Semiphore"=w443, "Expansion Tank?"=w442, "Valve Bank Setting"=ValveBankPositions."Heating", "Error In"=w446) -> ("Error Out"=w445:errorcluster)  [unwired: 9 in, 1 out]
                }
                frame Error {
                  n232 = Unbundle By Name(w450) -> ("source"=w455:string)
                  n233 = local read "FileName"() -> (w452:path)
                  n234 = Concatenate Strings("Error: " ("string"), w455) -> (w453:string)
                  n235 = call "String_in_Reference.vi"("String"=w453) -> ("String Out"=w451:string)  [unwired: 18 in]
                  n236 = call "Log String to Spreadsheet.vi"("String"=w451, "FileName"=w452) -> ()  [unwired: 9 in, 1 out]
                }
              }
            }
            frame "1." {
              # "30 minute delay after stability."
              n237 = call "E-Time.vi"("error in (no error)"=w459) -> ("error out"=w458:errorcluster, "Elapsed Time (sec)"=w457:dbl)  [unwired: 8 in, 1 out]
              n238 = while {
                tunnel: [w513] -> w464
                tunnel: w458 -> [w517]
                tunnel: [w510] -> w461
                tunnel: w457 -> [w506]
                stop <- w518 stop-if-true
                n239 = call "E-Time.vi"("error in (no error)"=w517) -> ("error out"=w512:errorcluster, "Elapsed Time (sec)"=w507:dbl)  [unwired: 8 in, 1 out]
                n240 = case shown="True" "1.SkipDelay" {
                  tunnel: [w521 w525] -> w513
                  tunnel: w512 -> [w521 w524]
                  frame False {
                  }
                  frame True {
                    n241 = local read "FileName"() -> (w522:path)
                    n242 = call "Log String to Spreadsheet.vi"("String"="30 Min Dealy Skipped", "error in (no error)"=w524, "FileName"=w522) -> ("error out"=w525:errorcluster)  [unwired: 8 in]
                  }
                }
                n243 = local read "Stop Logging"() -> (w510:bool)
                n244 = Subtract(x=w507, y=w506) -> (x-y=w508:dbl)
                n245 = Divide(x=w508, y=60.0) -> (x/y=w515:dbl)
                n246 = Subtract(x="Time Delay(30)", y=w515) -> (x-y=w514:dbl)
                "1.Delay Mins(30)" <- w514
                n247 = Less Or Equal To 0?(x=w514) -> (x <= 0?=w519:bool)
                n248 = local read "T1"() -> (w509:u32)
                n249 = Wait (ms)(milliseconds to wait=w509) -> ()  [unwired: 1 out]
                n250 = Compound Arithmetic op=OR(w519, "1.SkipDelay", w510) -> (w518:bool)
              }
              n251 = control-ref of="Downspout Temp"() -> (w460:refnum<vi>)
              n252 = local read "Test Condition"() -> (w463:T2)
              n253 = control-ref of="Downspout Flow Chart"() -> (w465:refnum<vi>)
              n254 = case shown="False" w461 {
                tunnel: w469 -> [w494 _]
                tunnel: [w477 w505] -> w468
                tunnel: [w493 _] -> w467
                tunnel: w466 -> [w475 _]
                tunnel: w465 -> [w492 _]
                tunnel: w464 -> [w489 w505]
                tunnel: w463 -> [w483 _]
                tunnel: [w482 _] -> w462
                tunnel: w460 -> [w481 _]
                frame False {
                  n255 = local read "FileName"() -> (w485:path)
                  n256 = flat-sequence {
                    tunnel: "PurgeBegins" ("string") -> [w504]
                    tunnel: w489 -> [w503]
                    tunnel: [w502] -> w488
                    tunnel: w485 -> [w501]
                    frame #0 {
                      n257 = call "String_in_Reference.vi"("String"=w504) -> ()  [unwired: 18 in, 1 out]
                      n258 = call "Log String to Spreadsheet.vi"("String"=w504, "error in (no error)"=w503, "FileName"=w501) -> ("error out"=w502:errorcluster)  [unwired: 8 in]
                    }
                  }
                  n259 = local read "Temp Band(+/- F)"() -> (w491:dbl)
                  n260 = call "Purge Water Sequence SM.vi"("Degree Setting"="Degree Setting", "Equipment"=w494, "Semiphore"=w475, "Flow rate setting"="Flow rate setting", "Temp Band(+/- F)"=w491, "Error In"=w488, "Flow Chart Ref"=w492, "Temp Chart Ref"=w481, "Test Condition"=w483) -> ("Flow rate setting out"=w493:dbl, "Temp Setting Out"=w482:dbl, "Error Out"=w487:errorcluster)  [unwired: 1 in, 3 out]
                  n261 = flat-sequence {
                    tunnel: w487 -> [w500]
                    tunnel: [w499] -> w486
                    tunnel: w485 -> [w498]
                    tunnel: "PurgeEnds" ("string") -> [w497]
                    frame #0 {
                      n262 = call "String_in_Reference.vi"("String"=w497) -> ()  [unwired: 18 in, 1 out]
                      n263 = call "Log String to Spreadsheet.vi"("String"=w497, "error in (no error)"=w500, "FileName"=w498) -> ("error out"=w499:errorcluster)  [unwired: 8 in]
                    }
                  }
                  n264 = local read "Expansion Tank?"() -> (w479:bool)
                  n265 = call <vilib>:"Clear Errors.vi"("error in (no error)"=w486) -> ("error out"=w473:errorcluster)  [unwired: 6 in]
                  n266 = local read "MW100"() -> (w476:refnum<visa-resource-name>)
                  n267 = call "HEWH Set Valves.vi"("VISA session"=w476, "Semiphore"=w475, "Expansion Tank?"=w479, "Valve Bank Setting"=ValveBankPositions."Draw", "Error In"=w473) -> ("Error Out"=w478:errorcluster)  [unwired: 9 in, 1 out]
                  n268 = call "HEWH Totalize Flow Control.vi"("VISA session"=w476, "Semiphore"=w475, "Totalize Flow"=TRUE, "error in (no error)"=w478) -> ("error out"=w477:errorcluster)  [unwired: 10 in, 1 out]
                }
                frame True {
                }
              }
              "Flowrate adj" <- w467
              "Temp adj" <- w462
              n269 = case shown="Error" w468 {
                selector: w468 -> [w526 w528]
                tunnel: [w527 string[] ["Finish"] ("States")] -> w471
                tunnel: w470 -> [w527 _]
                tunnel: [w526 w528] -> w472
                frame No Error {
                }
                frame Error {
                  n270 = Unbundle By Name(w528) -> ("source"=w533:string)
                  n271 = local read "FileName"() -> (w530:path)
                  n272 = Concatenate Strings("Error: " ("string"), w533) -> (w531:string)
                  n273 = call "String_in_Reference.vi"("String"=w531) -> ("String Out"=w529:string)  [unwired: 18 in]
                  n274 = call "Log String to Spreadsheet.vi"("String"=w529, "FileName"=w530) -> ()  [unwired: 9 in, 1 out]
                  "Error Out 1" <- w528
                }
              }
            }
            frame "2." {
              n275 = while {
                tunnel: [w565] -> w539
                tunnel: w536 -> [w594]
                shift-right: [w595] -> w540
                shift-left: w535 -> [w608]
                i -> [w600]
                stop <- w598 stop-if-true
                n276 = local read "Flow Adjust Time (3s)"() -> (w572:dbl)
                n277 = local read "Flow rate setting"() -> (w579:dbl)
                n278 = local read "Degree Setting"() -> (w578:dbl)
                n279 = local read "T2"() -> (w606:u32)
                n280 = local read "Serial Data In"() -> (w568:string)
                n281 = local read "Use Agilent?"() -> (w569:bool)
                n282 = local read "Label Array"() -> (w567:string[])
                n283 = local read "Equipment"() -> (w605:T7)
                n284 = local read "Chanel List"() -> (w604:string)
                n285 = local read "K(0.1)"() -> (w571:dbl)
                n286 = control-ref of="Tank Display"() -> (w603:refnum<vi>)
                n287 = Wait (ms)(milliseconds to wait=w606) -> ()  [unwired: 1 out]
                n288 = call "Gather Test Data - Heatup Test new.vi"("Agilent Scan List"=w604, "Semiphore"=w594, "Equipment"=w605, "Tank Display Ref"=w603, "Agilent?"=w569, "error in (no error)"=w608, "Serial Data In"=w568, "Agilent Label Array"=w567) -> ("Output Data"=w583:string[][], "POWER"=w609:T3, "Voltage"=w570:dbl, "error out"=w591:errorcluster)  [unwired: 2 in, 2 out]
                n289 = local read "Test Condition"() -> (w592:T2)
                n290 = local read "Temp adj"() -> (w574:dbl)
                n291 = local write "Voltage"(w570) -> ()
                n292 = local write "Test Data"(w583) -> ()
                n293 = local read "MW100"() -> (w593:refnum<visa-resource-name>)
                n294 = for {
                  tunnel: string[] ["GALLONS", "FLOW(GPM)", "Tc_down", "Board Address"] -> [w613] mode=indexing
                  tunnel: [w612] -> w585 mode=indexing
                  tunnel: w583 -> [w611]
                  n295 = call "Array_Search_For_Num.vi"("N Rows of Data"=w611, "Title?"=w613) -> ("number"=w612:dbl)  [unwired: 12 in, 1 out]
                }
                n296 = local write "POWER"(w609) -> ()
                n297 = call "E-Time.vi"("error in (no error)"=w591) -> ("error out"=w590:errorcluster, "Elapsed Time (sec)"=w589:dbl)  [unwired: 8 in, 1 out]
                n298 = local read "Flowrate adj"() -> (w575:dbl)
                n299 = Unbundle(w609) -> ("LE"=w563:bool, "COMP"=w566:bool, "FANS"=w597:bool)  [unwired: 1 out]
                n300 = Index Array(array=w585, index #1=0 ("index"), index #2=1 ("index"), index #3=2 ("index"), index #4=3 ("index")) -> (element #1=w582:dbl, element #2=w581:dbl, element #3=w580:dbl, element #4=w561:dbl)
                "2.TotWater" <- w582
                n301 = call "HEWH Flow Adjustment.vi"("VISA session"=w593, "Configuration"=w592, "Semiphore"=w594, "GPM Target(3)"=w579, "GPM reading"=w581, "Flow rate setting In"=w575, "Error In"=w590, "Elapsed Time (sec)"=w589, "Flow Adjust Time (3s)"=w572, "K(0.1)"=w571) -> ("Flow rate setting Out"=w576:dbl, "Error Out"=w596:errorcluster)  [unwired: 3 in, 1 out]
                n302 = Compound Arithmetic op=OR(w563, w566, w597) -> (w564:bool)
                n303 = local read "Stop Logging"() -> (w573:bool)
                n304 = call "HEWH Temp Adjustment.vi"("VISA session"=w593, "Semiphore"=w594, "Degrees Target(58)"=w578, "Degrees reading"=w580, "Degrees setting In"=w574, "Error In"=w596, "Elapsed Time (sec)"=w589, "Temp Adjust Time (3s)"=w572, "K(0.1)"=w571) -> ("Degree setting Out"=w577:dbl, "Error Out"=w595:errorcluster)  [unwired: 4 in, 1 out]
                n305 = Equal?(x=w561, y=256.0) -> (x = y?=w559:bool)
                n306 = Compound Arithmetic op=AND(invert w559, w564) -> (w565:bool)
                "2.Bottom Source Indicator" <- w565
                n307 = Greater Or Equal?(x=w582, y="2. Initial Draw") -> (x >= y?=w602:bool)
                n308 = Equal To 0?(x=w600) -> (x = 0?=w599:bool)
                n309 = Unbundle By Name(w595) -> ("status"=w607:bool)
                n310 = local write "Temp adj"(w577) -> ()
                n311 = local write "Flowrate adj"(w576) -> ()
                n312 = Compound Arithmetic op=OR(w607, w602, w565, w573) -> (w598:bool)
                n313 = Compound Arithmetic op=OR(w599, w598) -> (w601:bool)
                n314 = case shown="True" w601 {
                  tunnel: w583 -> [_ w614]
                  frame False {
                  }
                  frame True {
                    n315 = local read "FileName"() -> (w619:path)
                    n316 = Index Array(array=w614, index (row)=1) -> (element=w617:string[])  [unwired: 1 in]
                    n317 = call-poly <vilib>:"Write To Spreadsheet File.vi"("delimiter (\\t)"="," ("delimiter (\\t)"), "append to file? (new file:F)"=TRUE, "1D data"=w617, "file path (dialog if empty)"=w619) -> ()  [unwired: 4 in, 1 out]
                  }
                }
              }
              n318 = case shown="True" w539 {
                tunnel: [w553 w558] -> w541
                tunnel: w540 -> [w551 w558]
                tunnel: [w552 w557] -> w538
                tunnel: w537 -> [w552 w556]
                tunnel: w536 -> [w548 _]
                frame False {
                  n319 = local read "Expansion Tank?"() -> (w546:bool)
                  n320 = local read "MW100"() -> (w547:refnum<visa-resource-name>)
                  n321 = call "HEWH Set Valves.vi"("VISA session"=w547, "Semiphore"=w548, "Expansion Tank?"=w546, "Valve Bank Setting"=ValveBankPositions."Heating", "Error In"=w551) -> ("dup VISA session"=w549:refnum<visa-resource-name>, "Error Out"=w550:errorcluster)  [unwired: 9 in]
                  n322 = call "HEWH Totalize Flow Control.vi"("VISA session"=w549, "Semiphore"=w548, "Totalize Flow"=FALSE, "error in (no error)"=w550) -> ("error out"=w553:errorcluster)  [unwired: 10 in, 1 out]
                }
                frame True {
                  # "DELETE\n3,4."
                  n323 = Delete From Array(array=w556, length=2, index=0) -> (array with subset deleted=w557:string[])  [unwired: 1 out]
                }
              }
              n324 = case shown="Error" w541 {
                selector: w541 -> [w620 w622]
                tunnel: [w621 string[] ["Finish"] ("States")] -> w542
                tunnel: w538 -> [w621 _]
                tunnel: [w620 w622] -> w543
                frame No Error {
                }
                frame Error {
                  n325 = Unbundle By Name(w622) -> ("source"=w627:string)
                  n326 = local read "FileName"() -> (w624:path)
                  n327 = Concatenate Strings("Error: " ("string"), w627) -> (w625:string)
                  n328 = call "String_in_Reference.vi"("String"=w625) -> ("String Out"=w623:string)  [unwired: 18 in]
                  n329 = call "Log String to Spreadsheet.vi"("String"=w623, "FileName"=w624) -> ()  [unwired: 9 in, 1 out]
                }
              }
            }
            frame "3." {
              # "IS FLOW AND TEMP CONTROL NEEDED?"
              # "3.\tIf lower heat source does not energize during 10.75 gallon draw, then wait a maximum of 10 minutes to see if lower heat source will energize.  If it does, then allow the water heater to recover to set point."
              n330 = call "E-Time.vi"("error in (no error)"=w631) -> ("error out"=w632:errorcluster, "Elapsed Time (sec)"=w629:dbl)  [unwired: 8 in, 1 out]
              n331 = while {
                tunnel: [w697] -> w635
                shift-right: [w703] -> w634
                shift-left: w632 -> [w691]
                tunnel: w630 -> [w692]
                tunnel: w629 -> [w700]
                i -> [w683]
                stop <- w685 stop-if-true
                # "Continue to step 4."
                # "Stop when LE turns off"
                n332 = local read "Use Agilent?"() -> (w677:bool)
                n333 = local read "Serial Data In"() -> (w680:string)
                n334 = local read "Label Array"() -> (w679:string[])
                n335 = local read "T2"() -> (w698:u32)
                n336 = local read "Chanel List"() -> (w694:string)
                n337 = Wait (ms)(milliseconds to wait=w698) -> ()  [unwired: 1 out]
                n338 = local read "Equipment"() -> (w695:T7)
                n339 = control-ref of="Tank Display"() -> (w693:refnum<vi>)
                n340 = local read "Stop Logging"() -> (w681:bool)
                n341 = Equal To 0?(x=w683) -> (x = 0?=w684:bool)
                n342 = call "Gather Test Data - Heatup Test new.vi"("Agilent Scan List"=w694, "Semiphore"=w692, "Equipment"=w695, "Tank Display Ref"=w693, "Agilent?"=w677, "error in (no error)"=w691, "Serial Data In"=w680, "Agilent Label Array"=w679) -> ("Output Data"=w687:string[][], "POWER"=w690:T3, "Voltage"=w678:dbl, "error out"=w688:errorcluster)  [unwired: 2 in, 2 out]
                n343 = local write "POWER"(w690) -> ()
                n344 = local write "Voltage"(w678) -> ()
                n345 = Unbundle(w690) -> ("UE"=w672:bool, "LE"=w673:bool, "COMP"=w689:bool, "FANS"=w682:bool)
                n346 = local write "Test Data"(w687) -> ()
                n347 = call "E-Time.vi"("error in (no error)"=w688) -> ("error out"=w703:errorcluster, "Elapsed Time (sec)"=w701:dbl)  [unwired: 8 in, 1 out]
                n348 = And(x=w672, y=w673) -> (x .and. y?=w674:bool)
                n349 = Compound Arithmetic op=OR(w672, w673, w689, w682) -> (w675:bool)
                n350 = Subtract(x=w701, y=w700) -> (x-y=w699:dbl)
                n351 = Compound Arithmetic op=AND(invert w674, w675) -> (w676:bool)
                "3.Heat Source Indicator" <- w676
                n352 = Subtract(x="Wait Time(600s)", y=w699) -> (x-y=w696:dbl)
                "3.WaitTime(10min)" <- w696
                n353 = Less Or Equal To 0?(x=w696) -> (x <= 0?=w697:bool)
                n354 = Compound Arithmetic op=OR(w697, w676, w681) -> (w685:bool)
                n355 = Compound Arithmetic op=OR(w685, w684) -> (w686:bool)
                n356 = case shown="True" w686 {
                  tunnel: w687 -> [_ w704]
                  frame False {
                  }
                  frame True {
                    n357 = local read "FileName"() -> (w709:path)
                    n358 = Index Array(array=w704, index (row)=1) -> (element=w707:string[])  [unwired: 1 in]
                    n359 = call-poly <vilib>:"Write To Spreadsheet File.vi"("delimiter (\\t)"="," ("delimiter (\\t)"), "append to file? (new file:F)"=TRUE, "1D data"=w707, "file path (dialog if empty)"=w709) -> ()  [unwired: 4 in, 1 out]
                  }
                }
              }
              n360 = case shown="False" w635 {
                tunnel: w634 -> [w641 _]
                tunnel: [w640 errorcluster {"status"=TRUE, "code"=7003, "source"="FAIL!. Heating did not come on in time."} ("error out")] -> w633
                tunnel: w630 -> [w639 _]
                frame False {
                  n361 = while {
                    tunnel: w641 -> [w655]
                    tunnel: [w653] -> w640
                    tunnel: w639 -> [w654]
                    i -> [w650]
                    stop <- w648 continue-if-true
                    # "Recover."
                    n362 = local read "Use Agilent?"() -> (w645:bool)
                    n363 = local read "Chanel List"() -> (w657:string)
                    n364 = local read "Serial Data In"() -> (w643:string)
                    n365 = local read "Label Array"() -> (w642:string[])
                    n366 = control-ref of="Tank Display"() -> (w658:refnum<vi>)
                    n367 = Equal To 0?(x=w650) -> (x = 0?=w651:bool)
                    n368 = local read "Equipment"() -> (w656:T7)
                    n369 = call "Gather Test Data - Heatup Test new.vi"("Agilent Scan List"=w657, "Semiphore"=w654, "Equipment"=w656, "Tank Display Ref"=w658, "Agilent?"=w645, "error in (no error)"=w655, "Serial Data In"=w643, "Agilent Label Array"=w642) -> ("Output Data"=w649:string[][], "POWER"=w659:T3, "Voltage"=w644:dbl, "error out"=w653:errorcluster)  [unwired: 2 in, 2 out]
                    n370 = local write "POWER"(w659) -> ()
                    n371 = local read "Stop Logging"() -> (w646:bool)
                    n372 = local write "Test Data"(w649) -> ()
                    n373 = local write "Voltage"(w644) -> ()
                    n374 = Unbundle(w659) -> ("UE"=w660:bool, "LE"=w661:bool, "COMP"=w662:bool)  [unwired: 1 out]
                    n375 = local read "T2"() -> (w663:u32)
                    n376 = Compound Arithmetic op=OR(w660, w661, w662) -> (w647:bool)
                    n377 = Compound Arithmetic op=OR(invert w647, w651) -> (w652:bool)
                    n378 = case shown="True" w652 {
                      tunnel: w649 -> [_ w664]
                      frame False {
                      }
                      frame True {
                        n379 = local read "FileName"() -> (w669:path)
                        n380 = Index Array(array=w664, index (row)=1) -> (element=w667:string[])  [unwired: 1 in]
                        n381 = call-poly <vilib>:"Write To Spreadsheet File.vi"("delimiter (\\t)"="," ("delimiter (\\t)"), "append to file? (new file:F)"=TRUE, "1D data"=w667, "file path (dialog if empty)"=w669) -> ()  [unwired: 4 in, 1 out]
                      }
                    }
                    n382 = Wait (ms)(milliseconds to wait=w663) -> ()  [unwired: 1 out]
                    n383 = Compound Arithmetic op=AND(invert w646, w647) -> (w648:bool)
                  }
                }
                frame True {
                  n384 = local read "FileName"() -> (w670:path)
                  n385 = call "Log String to Spreadsheet.vi"("FileName"=w670) -> ()  [unwired: 10 in, 1 out]
                }
              }
              n386 = case shown="Error" w633 {
                selector: w633 -> [w710 w712]
                tunnel: [w711 string[] ["Finish"] ("States")] -> w637
                tunnel: w636 -> [w711 _]
                tunnel: [w710 w712] -> w638
                frame No Error {
                }
                frame Error {
                  n387 = Unbundle By Name(w712) -> ("source"=w717:string)
                  n388 = local read "FileName"() -> (w714:path)
                  n389 = Concatenate Strings("Error: " ("string"), w717) -> (w715:string)
                  n390 = call "String_in_Reference.vi"("String"=w715) -> ("String Out"=w713:string)  [unwired: 18 in]
                  n391 = call "Log String to Spreadsheet.vi"("String"=w713, "FileName"=w714) -> ()  [unwired: 9 in, 1 out]
                  "error 3" <- w712
                }
              }
            }
            frame "4." {
              # "4.\tAllow unit to sit 5 to 10 minutes in stabilized conditions, then:"
              n392 = disable-structure shown="Enabled" {
                disable-tunnel: w721 -> [w730 w731]
                disable-tunnel: [w729 w731] -> w720
                disable-tunnel: w719 -> [w728 _]
                frame Disabled {
                  n393 = local read "MW100"() -> (w727:refnum<visa-resource-name>)
                  n394 = call "YKMW100 Computation Control.vi"("VISA session"=w727, "Semiphore"=w728, "Mode"=T14."Reset Computation", "error in (no error)"=w730) -> ("error out"=w729:errorcluster)  [unwired: 10 in, 1 out]
                }
                frame Enabled {
                }
              }
              n395 = call "E-Time.vi"("error in (no error)"=w720) -> ("error out"=w725:errorcluster, "Elapsed Time (sec)"=w722:dbl)  [unwired: 8 in, 1 out]
              n396 = while {
                tunnel: w725 -> [w743]
                tunnel: [w741] -> w723
                tunnel: w722 -> [w734]
                stop <- w740 continue-if-true
                n397 = call "E-Time.vi"("error in (no error)"=w743) -> ("error out"=w741:errorcluster, "Elapsed Time (sec)"=w735:dbl)  [unwired: 8 in, 1 out]
                n398 = Subtract(x=w735, y=w734) -> (x-y=w733:dbl)
                n399 = local read "Stop Logging"() -> (w732:bool)
                n400 = Subtract(x="Delay(300s)", y=w733) -> (x-y=w742:dbl)
                "4.Delay Remaining (300s)" <- w742
                n401 = local read "T2"() -> (w737:u32)
                n402 = Greater Than 0?(x=w742) -> (x > 0?=w739:bool)
                n403 = Wait (ms)(milliseconds to wait=w737) -> ()  [unwired: 1 out]
                n404 = Compound Arithmetic op=AND(w739, invert "4.Skip Delay", invert w732) -> (w740:bool)
              }
            }
            frame "5." {
              n405 = local read "Flowrate adj"() -> (w758:dbl)
              n406 = local read "Temp adj"() -> (w754:dbl)
              n407 = local read "MW100"() -> (w749:refnum<visa-resource-name>)
              n408 = call "Solenoid Bank.vi"("VISA session"=w749, "Semiphore"=w748, "Drain Valve"=enum8{"OPEN", "CLOSE"}."CLOSE", "Output Valve"=enum8{"CLOSE", "OPEN"}."OPEN", "Input Valve"=enum8{"OPEN", "CLOSE"}."OPEN", "Error In"=w750) -> ("dup VISA session"=w747:refnum<visa-resource-name>, "Error Out"=w751:errorcluster)  [unwired: 8 in]
              n409 = call "HEWH Totalize Flow Control.vi"("VISA session"=w747, "Semiphore"=w748, "Totalize Flow"=TRUE, "error in (no error)"=w751) -> ("error out"=w753:errorcluster)  [unwired: 10 in, 1 out]
              n410 = while {
                shift-right: [w801] -> w760
                shift-left: w753 -> [w809]
                shift-right: [w821] -> w756
                shift-left: w758 -> [w822]
                tunnel: w748 -> [w792]
                tunnel: w764 -> [w819]
                tunnel: [w792] -> w759
                tunnel: [w817] -> w757
                shift-right: [w791] -> w755
                shift-left: w754 -> [w788]
                i -> [w805]
                stop <- w803 stop-if-true
                n411 = local read "Serial Data In"() -> (w784:string)
                n412 = local read "Use Agilent?"() -> (w782:bool)
                n413 = local read "Label Array"() -> (w783:string[])
                n414 = local read "T3"() -> (w816:u32)
                n415 = local read "Flow rate setting"() -> (w794:dbl)
                n416 = local read "Degree Setting"() -> (w795:dbl)
                n417 = local read "Chanel List"() -> (w812:string)
                n418 = local read "Equipment"() -> (w813:T7)
                n419 = Wait (ms)(milliseconds to wait=w816) -> ()  [unwired: 1 out]
                n420 = control-ref of="Tank Display"() -> (w811:refnum<vi>)
                n421 = call "Gather Test Data - Heatup Test new.vi"("Agilent Scan List"=w812, "Semiphore"=w792, "Equipment"=w813, "Tank Display Ref"=w811, "Agilent?"=w782, "error in (no error)"=w809, "Serial Data In"=w784, "Agilent Label Array"=w783) -> ("Output Data"=w797:string[][], "POWER"=w807:T3, "Voltage"=w785:dbl, "error out"=w808:errorcluster)  [unwired: 2 in, 2 out]
                n422 = local write "Voltage"(w785) -> ()
                n423 = local write "Test Data"(w797) -> ()
                n424 = local read "MW100"() -> (w806:refnum<visa-resource-name>)
                n425 = local write "POWER"(w807) -> ()
                n426 = call "E-Time.vi"("error in (no error)"=w808) -> ("error out"=w820:errorcluster, "Elapsed Time (sec)"=w799:dbl)  [unwired: 8 in, 1 out]
                n427 = call "Array_Search_For_Num.vi"("N Rows of Data"=w797, "Title?"="Tc_down") -> ("number"=w796:dbl)  [unwired: 12 in, 1 out]
                n428 = call "Array_Search_For_Num.vi"("N Rows of Data"=w797, "Title?"="FLOW(GPM)") -> ("number"=w810:dbl)  [unwired: 12 in, 1 out]
                "Downspout Flow" <- w810
                "Downspout Flow Chart" <- w810
                n429 = call "Array_Search_For_Num.vi"("N Rows of Data"=w797, "Title?"="GALLONS") -> ("number"=w780:dbl)  [unwired: 12 in, 1 out]
                "Total Gal Out" <- w780
                n430 = call "HEWH Flow Adjustment.vi"("VISA session"=w806, "Configuration"="Test Condition", "Semiphore"=w792, "GPM Target(3)"=w794, "GPM reading"=w810, "Flow rate setting In"=w822, "Error In"=w820, "Elapsed Time (sec)"=w799, "Flow Adjust Time (3s)"="Flow Adjust Time (3s)", "K(0.1)"="K(0.1)") -> ("VISA session out"=w793:refnum<visa-resource-name>, "Flow rate setting Out"=w821:dbl, "Error Out"=w800:errorcluster)  [unwired: 3 in]
                n431 = Equal To 0?(x=w805) -> (x = 0?=w802:bool)
                n432 = call "HEWH Temp Adjustment.vi"("VISA session"=w793, "Semiphore"=w792, "Degrees Target(58)"=w795, "Degrees reading"=w796, "Degrees setting In"=w788, "Error In"=w800, "Elapsed Time (sec)"=w799, "Temp Adjust Time (3s)"="Flow Adjust Time (3s)", "K(0.1)"="K(0.1)") -> ("Degree setting Out"=w791:dbl, "Error Out"=w801:errorcluster)  [unwired: 4 in, 1 out]
                n433 = case shown="Default" w819 {
                  tunnel: w780 -> [w830 _]
                  tunnel: [w829 w833] -> w817
                  tunnel: w807 -> [_ w834]
                  frame "E-Heat Mode" {
                    n434 = Greater Or Equal?(x=w830, y="Eheat Gal Limit") -> (x >= y?=w829:bool)
                  }
                  frame Default {
                    n435 = Unbundle(w834) -> ("UE"=w835:bool, "LE"=w832:bool)  [unwired: 2 out]
                    n436 = Compound Arithmetic op=AND(w835, invert w832) -> (w833:bool)
                  }
                }
                n437 = local read "Stop Logging"() -> (w789:bool)
                n438 = Greater Or Equal?(x=w780, y="Total Gal Limit") -> (x >= y?=w779:bool)
                n439 = Unbundle By Name(w801) -> ("status"=w818:bool)
                n440 = Compound Arithmetic op=OR(w779, w818, w817, w789) -> (w803:bool)
                n441 = Compound Arithmetic op=OR(w802, w803) -> (w804:bool)
                n442 = case shown="True" w804 {
                  tunnel: w797 -> [_ w823]
                  frame False {
                  }
                  frame True {
                    n443 = local read "FileName"() -> (w828:path)
                    n444 = Index Array(array=w823, index (row)=1) -> (element=w826:string[])  [unwired: 1 in]
                    n445 = call-poly <vilib>:"Write To Spreadsheet File.vi"("delimiter (\\t)"="," ("delimiter (\\t)"), "append to file? (new file:F)"=TRUE, "1D data"=w826, "file path (dialog if empty)"=w828) -> ()  [unwired: 4 in, 1 out]
                  }
                }
              }
              "5.Top Source Indicator" <- w757
              n446 = case shown="No Error" w760 {
                selector: w760 -> [w770 w772]
                tunnel: [w771 string[] ["Finish"] ("States")] -> w762
                tunnel: w763 -> [w771 _]
                tunnel: [w767 w772] -> w761
                tunnel: w759 -> [w768 _]
                frame No Error {
                  n447 = local read "Expansion Tank?"() -> (w766:bool)
                  n448 = local read "MW100"() -> (w769:refnum<visa-resource-name>)
                  n449 = call "HEWH Set Valves.vi"("VISA session"=w769, "Semiphore"=w768, "Expansion Tank?"=w766, "Valve Bank Setting"=ValveBankPositions."Heating", "Error In"=w770) -> ("Error Out"=w767:errorcluster)  [unwired: 9 in, 1 out]
                }
                frame Error {
                  n450 = Unbundle By Name(w772) -> ("source"=w777:string)
                  n451 = local read "FileName"() -> (w774:path)
                  n452 = Concatenate Strings("Error: " ("string"), w777) -> (w775:string)
                  n453 = call "String_in_Reference.vi"("String"=w775) -> ("String Out"=w773:string)  [unwired: 18 in]
                  n454 = call "Log String to Spreadsheet.vi"("String"=w773, "FileName"=w774) -> ()  [unwired: 9 in, 1 out]
                  "Error 5" <- w772
                }
              }
              n455 = local write "Flowrate adj"(w756) -> ()
              n456 = local write "Temp adj"(w755) -> ()
            }
            frame "6." {
              # "6.\tIn Hybrid Mode: when the Upper Element stops and switches to Lower Element, switch the unit to eHeat Mode.  This will switch the lower heating source to Compressor."
              n457 = case shown="\"Hybrid Heating\"" w837 {
                tunnel: w840 -> [_ w844]
                tunnel: w839 -> [w843 w845]
                tunnel: [w843 w846] -> w838
                frame Default {
                }
                frame "Hybrid Heating" {
                  n458 = while {
                    tunnel: w844 -> [w869]
                    shift-right: [w874] -> w846
                    shift-left: w845 -> [_]
                    i -> [w856]
                    stop <- w862 stop-if-true
                    # "Sample the beginning and end."
                    n459 = local read "Use Agilent?"() -> (w864:bool)
                    n460 = local read "Serial Data In"() -> (w865:string)
                    n461 = local read "Label Array"() -> (w866:string[])
                    n462 = local read "T2"() -> (w847:u32)
                    n463 = local read "Chanel List"() -> (w871:string)
                    n464 = Wait (ms)(milliseconds to wait=w847) -> ()  [unwired: 1 out]
                    n465 = local read "Equipment"() -> (w872:T7)
                    n466 = control-ref of="Tank Display"() -> (w870:refnum<vi>)
                    n467 = local read "Stop Logging"() -> (w853:bool)
                    n468 = Equal To 0?(x=w856) -> (x = 0?=w855:bool)
                    n469 = call "Gather Test Data - Heatup Test new.vi"("Agilent Scan List"=w871, "Semiphore"=w869, "Equipment"=w872, "Tank Display Ref"=w870, "Agilent?"=w864, "Serial Data In"=w865, "Agilent Label Array"=w866) -> ("Output Data"=w868:string[][], "POWER"=w873:T3, "Voltage"=w863:dbl, "error out"=w867:errorcluster)  [unwired: 3 in, 2 out]
                    n470 = local write "Voltage"(w863) -> ()
                    n471 = local write "POWER"(w873) -> ()
                    n472 = local read "GEA2 HyperData"() -> (w859:bool)
                    n473 = local write "Test Data"(w868) -> ()
                    n474 = Unbundle(w873) -> ("UE"=w850:bool, "LE"=w851:bool, "COMP"=w848:bool)  [unwired: 1 out]
                    n475 = Compound Arithmetic op=AND(invert w850, w851) -> (w849:bool)
                    n476 = Or(x=w849, y=w848) -> (x .or. y?=w857:bool)
                    "6.Bottom Source Indicator" <- w857
                    n477 = Compound Arithmetic op=OR(w857, w855) -> (w854:bool)
                    n478 = Compound Arithmetic op=AND(w854, invert w853) -> (w852:bool)
                    n479 = case shown="True" w852 {
                      tunnel: w868 -> [_ w924]
                      frame False {
                      }
                      frame True {
                        n480 = local read "FileName"() -> (w923:path)
                        n481 = Index Array(array=w924, index (row)=1) -> (element=w921:string[])  [unwired: 1 in]
                        n482 = call-poly <vilib>:"Write To Spreadsheet File.vi"("delimiter (\\t)"="," ("delimiter (\\t)"), "append to file? (new file:F)"=TRUE, "1D data"=w921, "file path (dialog if empty)"=w923) -> ()  [unwired: 4 in, 1 out]
                      }
                    }
                    n483 = local read "FileName"() -> (w860:path)
                    n484 = case shown="True" w859 {
                      tunnel: [w880 w898] -> w874
                      tunnel: w869 -> [w879 w897]
                      tunnel: w857 -> [w878 w896]
                      tunnel: w867 -> [w877 w895]
                      tunnel: [w875 w894] -> w861
                      tunnel: w860 -> [w876 w893]
                      tunnel: [w875 w892] -> w858
                      frame False {
                        n485 = case shown="True" w878 {
                          tunnel: [FALSE ("true") TRUE ("true")] -> w875
                          tunnel: w877 -> [w882 w890]
                          tunnel: [w882 w884] -> w880
                          tunnel: w879 -> [_ w888]
                          tunnel: w876 -> [_ w883]
                          frame False {
                          }
                          frame True {
                            w887 = T6 2 items=["CRITICAL", "HIGH", "MEDIUM", "Normal"] ("Mode")
                            n486 = local read "MW100"() -> (w889:refnum<visa-resource-name>)
                            n487 = call "HEWH Set DRM Mode.vi"("MW100"=w889, "Semiphore"=w888, "Mode"=w887, "error in (no error)"=w890) -> ("error out"=w886:errorcluster)  [unwired: 11 in]
                            n488 = call "Log String to Spreadsheet.vi"("String"="Set Mode to Medium", "error in (no error)"=w886, "FileName"=w883) -> ("error out"=w884:errorcluster)  [unwired: 8 in]
                          }
                        }
                      }
                      frame True {
                        n489 = case shown="True" w896 {
                          tunnel: [w899 w903] -> w894
                          tunnel: w895 -> [w900 _]
                          tunnel: [w900 w918] -> w898
                          tunnel: w897 -> [_ _]
                          tunnel: w893 -> [_ w917]
                          tunnel: [w899 w907] -> w892
                          frame False {
                            w899 = FALSE ("true")
                          }
                          frame True {
                            w912 = HEWH_Mode."eHeat" ("Mode")
                            n490 = local read "GEA2"() -> (w906:T1)
                            n491 = call "Counter.vi"() -> ("Count"=w909:dbl)  [unwired: 11 in]
                            n492 = local read "COM Port"() -> (w913:refnum<visa-resource-name>)
                            n493 = call <vilib>:"Acquire Semaphore.vi"("semaphore"=w906) -> ("error out"=w916:errorcluster, "semaphore out"=w915:T1)  [unwired: 4 in, 1 out]
                            n494 = Greater?(x=w909, y=3.0) -> (0:w907:bool)
                            n495 = call "GEA2_CMD_UPDATE_MODE.vi"("ComPort"=w913, "Mode"=w912, "Error In"=w916) -> ("Error Out"=w901:errorcluster)  [unwired: 10 in, 2 out]
                            n496 = call "GEA2_RQST_STATUS_QUERY.vi"("ComPort"=w913, "Error In"=w901) -> ("Mode"=w911:T9, "Error Out"=w910:errorcluster)  [unwired: 8 in, 4 out]
                            n497 = Equal?(x=w912, y=w911) -> (x = y?=w903:bool)
                            n498 = call <vilib>:"Release Semaphore.vi"("error in (no error)"=w910, "semaphore"=w915) -> ("error out"=w914:errorcluster)  [unwired: 4 in, 1 out]
                            n499 = Select(t="Set Mode to eHeat" ("String"), s=w903, f="Fail Set Mode to eHeat" ("String")) -> (s? t:f=w902:string)
                            n500 = call "Log String to Spreadsheet.vi"("String"=w902, "error in (no error)"=w914, "FileName"=w917) -> ("error out"=w918:errorcluster)  [unwired: 8 in]
                          }
                        }
                      }
                    }
                    n501 = Compound Arithmetic op=OR(w861, w853, w858) -> (w862:bool)
                  }
                }
              }
              n502 = case shown="Error" w838 {
                selector: w838 -> [w925 w928]
                tunnel: [w926 string[] ["Finish"] ("States")] -> w842
                tunnel: w836 -> [w926 _]
                tunnel: [w925 w928] -> w841
                frame No Error {
                }
                frame Error {
                }
              }
            }
            frame "7." {
              # "7.\tAllow water heater to stabilize this second time. (Recover water temperature back to set point)."
              n503 = while {
                tunnel: w932 -> [w957]
                tunnel: w931 -> [w956]
                tunnel: [w958] -> w930
                i -> [w951]
                stop <- w950 continue-if-true
                n504 = local read "Use Agilent?"() -> (w945:bool)
                n505 = local read "Serial Data In"() -> (w948:string)
                n506 = local read "Label Array"() -> (w947:string[])
                n507 = local read "Chanel List"() -> (w960:string)
                n508 = Equal To 0?(x=w951) -> (x = 0?=w952:bool)
                n509 = local read "Stop Logging"() -> (w944:bool)
                n510 = local read "Equipment"() -> (w961:T7)
                n511 = control-ref of="Tank Display"() -> (w959:refnum<vi>)
                n512 = call "Gather Test Data - Heatup Test new.vi"("Agilent Scan List"=w960, "Semiphore"=w956, "Equipment"=w961, "Tank Display Ref"=w959, "Agilent?"=w945, "error in (no error)"=w957, "Serial Data In"=w948, "Agilent Label Array"=w947) -> ("Output Data"=w943:string[][], "POWER"=w962:T3, "Voltage"=w946:dbl, "error out"=w958:errorcluster)  [unwired: 2 in, 2 out]
                n513 = local write "POWER"(w962) -> ()
                n514 = local write "Voltage"(w946) -> ()
                n515 = local write "Test Data"(w943) -> ()
                n516 = Unbundle(w962) -> ("UE"=w935:bool, "LE"=w936:bool, "COMP"=w955:bool, "FANS"=w949:bool)
                n517 = local read "Tank Display"() -> (w942:T4)
                n518 = Compound Arithmetic op=AND(w935, w936) -> (invert w933:bool)
                n519 = Compound Arithmetic op=OR(w935, w936, w955, w949) -> (w939:bool)
                n520 = And(x=w933, y=w939) -> (x .and. y?=w934:bool)
                "7.Heat Source Indicator" <- w934
                n521 = Unbundle By Name(w942) -> ("Mean"=w941:dbl)
                "Mean Tank Temp" <- w941
                n522 = Less?(x=w941, y="Min Ave Temp Limit") -> (x < y?=w938:bool)
                n523 = Or(x=w938, y=w934) -> (x .or. y?=w937:bool)
                n524 = Compound Arithmetic op=AND(w937, invert "Skip Waiting for Bottom Source to turn off.", invert w944) -> (w950:bool)
                n525 = Compound Arithmetic op=OR(invert w950, w952) -> (w953:bool)
                n526 = Compound Arithmetic op=AND(w953, invert w944) -> (w954:bool)
                n527 = case shown="True" w954 {
                  tunnel: w943 -> [_ w970]
                  frame False {
                  }
                  frame True {
                    n528 = local read "FileName"() -> (w969:path)
                    n529 = Index Array(array=w970, index (row)=1) -> (element=w967:string[])  [unwired: 1 in]
                    n530 = call-poly <vilib>:"Write To Spreadsheet File.vi"("delimiter (\\t)"="," ("delimiter (\\t)"), "append to file? (new file:F)"=TRUE, "1D data"=w967, "file path (dialog if empty)"=w969) -> ()  [unwired: 4 in, 1 out]
                  }
                }
                n531 = local read "T2"() -> (w963:u32)
                n532 = Wait (ms)(milliseconds to wait=w963) -> ()  [unwired: 1 out]
              }
            }
            frame "8." {
              n533 = call "E-Time.vi"("error in (no error)"=w975) -> ("error out"=w973:errorcluster, "Elapsed Time (sec)"=w971:dbl)  [unwired: 8 in, 1 out]
              n534 = while {
                shift-right: [w986] -> w974
                shift-left: w973 -> [w987]
                tunnel: w971 -> [w981]
                stop <- w979 continue-if-true
                # "8.\tAllow unit to sit a minimum of 30 minutes in stabilized conditions, then;"
                n535 = local read "T2"() -> (w984:u32)
                n536 = call "E-Time.vi"("error in (no error)"=w987) -> ("error out"=w986:errorcluster, "Elapsed Time (sec)"=w982:dbl)  [unwired: 8 in, 1 out]
                n537 = Wait (ms)(milliseconds to wait=w984) -> ()  [unwired: 1 out]
                n538 = Subtract(x=w982, y=w981) -> (x-y=w980:dbl)
                n539 = Subtract(x="8.Delay(1800s)", y=w980) -> (x-y=w985:dbl)
                "Seconds to Completion" <- w985
                n540 = local read "Stop Logging"() -> (w978:bool)
                n541 = Greater Than 0?(x=w985) -> (x > 0?=w976:bool)
                n542 = Compound Arithmetic op=AND(w976, invert "8.Skip Waiting", invert w978) -> (w979:bool)
              }
            }
            frame "9." {
              w988 = T6 3 items=["CRITICAL", "HIGH", "MEDIUM", "Normal"] ("Mode")
              # "(Set DRM back to Normal)"
              # "9.\tStop Data Logger and HyperTerminal session."
              n543 = local read "MW100"() -> (w990:refnum<visa-resource-name>)
              n544 = local read "Semiphore"() -> (w989:T1)
              n545 = call "HEWH Set DRM Mode.vi"("MW100"=w990, "Semiphore"=w989, "Mode"=w988, "error in (no error)"=w992) -> ("error out"=w991:errorcluster)  [unwired: 11 in]
            }
            frame "Finish", Default {
              # "Stop Serail Data"
              # "Wait till logging loop completes"
              n546 = call "YKMW100 Get Error Log.vi"("Semiphore"=w997, "error in (no error)"=w998) -> ("dup VISA session"=w1000:refnum<visa-resource-name>, "Error History"=→"Error History":string[], "error out"=w1001:errorcluster)  [unwired: 10 in, 1 out]
              n547 = flat-sequence {
                tunnel: w1001 -> [w1008]
                tunnel: w1000 -> [w1007]
                tunnel: w997 -> [w1005]
                tunnel: [w1004] -> w995
                frame #0 {
                  w1003 = TRUE ("Stop Logging")
                  n548 = call "YKMW100 Get Com Log.vi"("VISA session"=w1007, "Semiphore"=w1005, "error in (no error)"=w1008) -> ("Com History"=→"Com History":string[], "error out"=w1004:errorcluster)  [unwired: 9 in, 2 out]
                  n549 = local write "Stop Logging"(w1003) -> ()
                  n550 = property on="Stop Logging" class="Bool (strict)"("Val(Sgnl)"=w1003) -> ()  [unwired: 2 in, 2 out]
                }
              }
              n551 = while {
                tunnel: [TRUE ("Stop Logging")] -> w996
                tunnel: [w1009] -> w994
                tunnel: w995 -> [w1009]
                stop <- w1012 stop-if-true
                n552 = local read "T1"() -> (w1011:u32)
                n553 = local read "St.Logging"() -> (w1012:bool)
                n554 = Wait (ms)(milliseconds to wait=w1011) -> ()  [unwired: 1 out]
              }
              n555 = case shown="True" w996 {
                tunnel: w994 -> [_ _]
                frame False {
                }
                frame True {
                  w1013 = TRUE
                  n556 = local write "StopSerial"(w1013) -> ()
                  n557 = property on="StopSerial" class="Bool (strict)"("Val(Sgnl)"=w1013) -> ()  [unwired: 2 in, 2 out]
                  "LoggingStopped" <- w1013
                }
              }
            }
          }
          n558 = Equal?(x=w218, y="Finish") -> (x = y?=w217:bool)
        }
        n559 = while {
          tunnel: w207 -> [w1026]
          shift-right: [w1022] -> _
          shift-left: 0.0 -> [w1019]
          i -> [w1025]
          stop <- w1024 stop-if-true
          # "continuous data gathering"
          n560 = local read "T4"() -> (w1014:i32)
          n561 = Multiply(x=w1019, y=1000.0) -> (x*y=w1021:dbl)
          n562 = To Long Integer(number=w1021) -> (32bit integer=w1018:i32)
          n563 = Subtract(x=w1014, y=w1018) -> (x-y=w1015:i32)
          n564 = In Range and Coerce(upper limit=w1014, x=w1015, lower limit=0) -> (coerced(x)=w1017:i32)  [unwired: 1 out]
          n565 = event shown="[0] Timeout" {
            selector: _ -> [_ _]
            dyn-events: _ -> [_ _]
            timeout: w1017 -> [_ _]
            tunnel: w1026 -> [w1072 _]
            tunnel: ["Stop Logging" TRUE ("Stop Logging")] -> w1024
            tunnel: [w1039 _] -> w1023
            event Timeout {
              n566 = event-data() -> ()  [unwired: 1 in, 2 out]
              n567 = local read "Use Agilent?"() -> (w1041:bool)
              n568 = local read "Serial Data In"() -> (w1042:string)
              n569 = local read "Chanel List"() -> (w1067:string)
              n570 = flat-sequence {
                tunnel: [w1084] -> w1040
                tunnel: [w1083] -> w1039
                frame #0 {
                  n571 = local read "Label Array"() -> (w1084:string[])
                  n572 = call "E-Time.vi"() -> ("Elapsed Time (sec)"=w1083:dbl)  [unwired: 9 in, 2 out]
                }
              }
              n573 = control-ref of="Tank Display"() -> (w1070:refnum<vi>)
              n574 = local read "Equipment"() -> (w1071:T7)
              n575 = call "Gather Test Data - Heatup Test new.vi"("Agilent Scan List"=w1067, "Semiphore"=w1072, "Equipment"=w1071, "Tank Display Ref"=w1070, "Agilent?"=w1041, "Serial Data In"=w1042, "Agilent Label Array"=w1040) -> ("Tc Tree"=w1046:dbl[], "Output Data"=w1065:string[][], "POWER"=w1064:T3, "PowerData"=w1069:T17, "Voltage"=w1038:dbl, "error out"=w1044:errorcluster)  [unwired: 3 in]
              "error datalogging" <- w1044
              n576 = local write "Voltage"(w1038) -> ()
              n577 = Unbundle By Name(w1069) -> ("Power"=w1060:dbl)
              "Watts" <- w1060
              n578 = call <vilib>:"Mean.vi"("X"=w1046) -> ("mean"=→"Ave Temp":dbl)  [unwired: 1 out]
              n579 = Array To Cluster(array=w1046) -> (cluster=w1068:T18)
              n580 = Unbundle(w1064) -> ("UE"=w1063:bool, "LE"=w1061:bool, "COMP"=w1062:bool, "FANS"=w1057:bool)
              n581 = Build Array(w1068) -> (→"Temps":T10)
              n582 = Boolean To (0,1)(Boolean=w1063) -> (0, 1=w1052:i16)
              n583 = Boolean To (0,1)(Boolean=w1062) -> (0, 1=w1050:i16)
              n584 = Boolean To (0,1)(Boolean=w1057) -> (0, 1=w1056:i16)
              n585 = Boolean To (0,1)(Boolean=w1061) -> (0, 1=w1051:i16)
              n586 = expression code="4*x"(w1052) -> (w1053:i16)
              n587 = expression code="3*x"(w1051) -> (w1054:i16)
              n588 = expression code="2*x"(w1050) -> (w1055:i16)
              n589 = call "Array_Search_For_Num.vi"("N Rows of Data"=w1065, "Title?"="GALLONS") -> ("number"=→"Gallons Chart" →"Gallons":dbl)  [unwired: 12 in, 1 out]
              n590 = Build Array(w1060, w1053, w1054, w1055, w1056) -> (w1058:dbl[])
              n591 = Unbundle By Name(w1044) -> ("status"=w1037:bool, "code"=w1035:i32, "source"=w1036:string)
              n592 = Array To Cluster(array=w1058) -> (cluster=w1059:T19)
              n593 = local write "Test Data"(w1065) -> ()
              n594 = Build Array(w1059) -> (→"Watt Chart":T11)
              n595 = Number To Decimal String(number=w1035) -> (decimal integer string=w1034:string)  [unwired: 1 in]
              n596 = case shown="True" w1037 {
                tunnel: w1036 -> [_ w1081]
                tunnel: w1034 -> [_ w1080]
                tunnel: "Error Datalog: " ("string") -> [_ w1079]
                tunnel: [_ w1079] -> w1032
                tunnel: [FALSE w1074] -> w1030
                frame False {
                }
                frame True {
                  n597 = call "Counter.vi"() -> ("Count"=w1076:dbl)  [unwired: 11 in]
                  n598 = local read "FileName"() -> (w1078:path)
                  n599 = Concatenate Strings(w1079, w1080, " " ("string"), w1081) -> (w1077:string)
                  n600 = Greater?(x=w1076, y="Com Err Limit") -> (0:w1074:bool)
                  n601 = call "Log String to Spreadsheet.vi"("String"=w1077, "FileName"=w1078) -> ()  [unwired: 9 in, 1 out]
                }
              }
              n602 = Compound Arithmetic op=OR("Stop Logging", w1030) -> (w1043:bool)
              n603 = case shown="True" w1043 {
                selector: w1043 -> [_ w1093]
                tunnel: w1065 -> [w1086 _]
                tunnel: w1032 -> [_ _]
                frame False {
                  n604 = local read "FileName"() -> (w1090:path)
                  n605 = Index Array(array=w1086, index (row)=1) -> (element=w1088:string[])  [unwired: 1 in]
                  n606 = call-poly <vilib>:"Write To Spreadsheet File.vi"("delimiter (\\t)"="," ("delimiter (\\t)"), "append to file? (new file:F)"=TRUE, "1D data"=w1088, "file path (dialog if empty)"=w1090) -> ()  [unwired: 4 in, 1 out]
                }
                frame True {
                  n607 = local read "FileName"() -> (w1092:path)
                  n608 = local write "Stop Logging"(w1093) -> ()
                  n609 = property on="Stop Logging" class="Bool (strict)"("Val(Sgnl)"=w1093) -> ()  [unwired: 2 in, 2 out]
                  n610 = call "Log String to Spreadsheet.vi"("String"="Stop Logging", "FileName"=w1092) -> ()  [unwired: 9 in, 1 out]
                  "St.Logging" <- w1093
                }
              }
            }
            event "Stop Logging": Value Change {
              n611 = event-data() -> ()  [unwired: 1 in, 5 out]
              n612 = local write "St.Logging"(TRUE ("St.Logging")) -> ()
            }
          }
          n613 = flat-sequence {
            tunnel: w1023 -> [w1028]
            tunnel: [w1027] -> w1022
            frame #0 {
              n614 = call "E-Time.vi"() -> ("Elapsed Time (sec)"=w1029:dbl)  [unwired: 9 in, 2 out]
              n615 = Subtract(x=w1029, y=w1028) -> (x-y=w1027:dbl)
            }
          }
          "Number of Records" <- w1025
        }
      }
      frame "Finish", Default {
        w1096 = TRUE
        n616 = local write "StopSerial"(w1096) -> ()
        n617 = property on="StopSerial" class="Bool (strict)"("Val(Sgnl)"=w1096) -> ()  [unwired: 2 in, 2 out]
        n618 = property on="Init Complete" class="Bool (strict)"("Val(Sgnl)"=w1096) -> ()  [unwired: 2 in, 2 out]
        n619 = case shown="Error" w1098 {
          selector: w1098 -> [w1103 w1110]
          tunnel: [w1104 string[] ["Finish"] ("States")] -> w1100
          tunnel: w1101 -> [w1104 _]
          tunnel: [w1103 w1110] -> w1102
          frame No Error {
          }
          frame Error {
            n620 = Unbundle By Name(w1110) -> ("source"=w1105:string)
            n621 = local read "FileName"() -> (w1108:path)
            n622 = Concatenate Strings("Error: " ("string"), w1105) -> (w1107:string)
            n623 = call "String_in_Reference.vi"("String"=w1107) -> ("String Out"=w1109:string)  [unwired: 18 in]
            n624 = call "Log String to Spreadsheet.vi"("String"=w1109, "FileName"=w1108) -> ()  [unwired: 9 in, 1 out]
          }
        }
      }
    }
    n625 = Equal?(x=w24, y="Finish") -> (x = y?=w31:bool)
  }
  "Error Out" <- w10
  n626 = event shown="[1] \"Init Complete\": Value Change" {
    selector: _ -> [_ _]
    dyn-events: _ -> [_ _]
    timeout: _ -> [_ _]
    tunnel: [_ w1114] -> w6
    tunnel: [_ w1113] -> w5
    tunnel: w1 -> [_ w1112]
    event Timeout {
      n627 = event-data() -> ()  [unwired: 1 in, 2 out]
    }
    event "Init Complete": Value Change {
      # "reading serial port"
      n628 = event-data() -> ()  [unwired: 1 in, 5 out]
      n629 = while {
        tunnel: ["StopSerial"] -> w1114
        tunnel: w1112 -> [w1121]
        tunnel: [w1118] -> w1113
        stop <- "StopSerial" stop-if-true
        n630 = flat-sequence {
          frame #0 {
            n631 = Wait (ms)(milliseconds to wait="mS Between Serial Polls") -> ()  [unwired: 1 out]
          }
        }
        n632 = local read "GEA2 HyperData"() -> (w1117:bool)
        n633 = local read "COM Port"() -> (w1127:refnum<visa-resource-name>)
        n634 = Select(t=10, s=w1117, f=1) -> (s? t:f=w1123:i32)
        n635 = call <vilib>:"Acquire Semaphore.vi"("semaphore"=w1121) -> ("error out"=w1122:errorcluster, "semaphore out"=w1119:T1)  [unwired: 4 in, 1 out]
        n636 = call "HEWH Serial Data Read.vi"("Serial Port Ref"=w1127, "GEA2 HyperData"=w1117, "Retries"=w1123, "error in (no error)"=w1122) -> ("Serial Read OK"=→"Serial Read OK":bool, "Read String"=w1129:string, "Retries"=→"Retries":i32, "error out"=w1128:errorcluster)  [unwired: 8 in]
        n637 = local write "Serial Data In"(w1129) -> ()
        n638 = call <vilib>:"Release Semaphore.vi"("error in (no error)"=w1128, "semaphore"=w1119) -> ("error out"=→"Error Serial":errorcluster, "semaphore out"=w1118:T1)  [unwired: 4 in]
      }
    }
  }
  n639 = flat-sequence {
    tunnel: w6 -> [_]
    tunnel: w5 -> [w1131]
    frame #0 {
      w1132 = TRUE ("stop")
      n640 = call <vilib>:"Release Semaphore Reference.vi"("semaphore"=w1131) -> ()  [unwired: 9 in, 2 out]
      n641 = property on="Stop" class="Bool (strict)"("Val(Sgnl)"=w1132) -> ()  [unwired: 2 in, 2 out]
      n642 = local write "Stop"(w1132) -> ()
      n643 = call "String_in_Reference.vi"("String"="Stopping Test") -> ()  [unwired: 18 in, 1 out]
    }
  }
  n644 = while {
    stop <- w1135 stop-if-true
    # "stop and help events"
    n645 = local read "T2"() -> (w1134:u32)
    n646 = event shown="[1] \"Stop\": Value Change" {
      selector: _ -> [_ _ _]
      dyn-events: _ -> [_ _ _]
      timeout: w1134 -> [_ _ _]
      tunnel: [FALSE ("stop? (T)") w1139 FALSE ("stop? (T)")] -> w1135
      event Timeout {
        n647 = event-data() -> ()  [unwired: 1 in, 2 out]
        n648 = call "E-Time.vi"() -> ("Elapsed Time (sec)"=→"Elapsed Time":dbl)  [unwired: 9 in, 2 out]
        n649 = call "String_in_Reference.vi"() -> ("String Out"=→"HEATUP TEST STATUS":string)  [unwired: 19 in]
      }
      event "Stop": Value Change {
        n650 = event-data() -> ()  [unwired: 1 in, 5 out]
        n651 = case shown="True" "Stop" {
          tunnel: [FALSE ("stop? (T)") w1142] -> w1139
          frame False {
          }
          frame True {
            n652 = stacked-sequence {
              tunnel: [_ _ _ _ TRUE ("stop? (T)") _] -> w1142
              frame #0 {
                # "Open outlet valve."
                n653 = local read "Semiphore"() -> (w1146:T1)
                n654 = local read "MW100"() -> (w1144:refnum<visa-resource-name>)
                n655 = local read "Expansion Tank?"() -> (w1143:bool)
                n656 = call "HEWH Set Valves.vi"("VISA session"=w1144, "Semiphore"=w1146, "Expansion Tank?"=w1143, "Valve Bank Setting"=ValveBankPositions."Resting") -> ()  [unwired: 10 in, 2 out]
              }
              frame #1 {
                n657 = local read "Local?"() -> (w1147:bool)
                n658 = case shown="True" w1147 {
                  tunnel: w1147 -> [_ w1148]
                  frame False {
                  }
                  frame True {
                    n659 = local read "Equipment"() -> (w1151:T7)
                    n660 = local read "Semiphore"() -> (w1150:T1)
                    n661 = call "HEWH CloseEquipmet.vi"("Semiphore"=w1150, "Equipment"=w1151) -> ("Error Out"=w1149:errorcluster)  [unwired: 9 in]
                    n662 = call "Semiphore-Destroy-Local.vi"("Semiphore"=w1150, "Local?"=w1148, "error in (no error)"=w1149) -> ()  [unwired: 16 in, 1 out]
                  }
                }
              }
              frame #2 {
                n663 = local read "FileName"() -> (w1152:path)
                n664 = local read "Init Complete"() -> (w1154:bool)
                n665 = call <vilib>:"Check if File or Folder Exists.vi"("path"=w1152) -> ("file or folder exists?"=w1155:bool)  [unwired: 8 in, 2 out]
                n666 = And(x=w1155, y=w1154) -> (x .and. y?=w1153:bool)
                n667 = case shown="True" w1153 {
                  tunnel: w1152 -> [_ w1163]
                  frame False {
                  }
                  frame True {
                    n668 = Strip Path(path=w1163) -> (name=w1162:string)  [unwired: 1 out]
                    n669 = Search and Replace String(input string=w1162, search string=".tmp", replace string=".csv" ("search string")) -> (result string=w1160:string, error out=w1166:errorcluster)  [unwired: 5 in, 2 out]
                    n670 = Build Path(base path="Save File Directory", name or relative path=w1160) -> (appended path=w1159:path)
                    n671 = Move(source path=w1163, error in=w1166, 10:w1159) -> (error out=w1158:errorcluster, 3:w1157:path)  [unwired: 2 in, 1 out]
                    n672 = Set Permissions(7:i16 0 ("permissions"), 8:w1158, 11:w1157) -> ()  [unwired: 2 in, 2 out]
                  }
                }
              }
              frame #3 {
                n673 = local write "Stop"(FALSE ("stop")) -> ()
                n674 = local write "HEATUP TEST STATUS"("Complete OK" ("STATUS")) -> ()
              }
              frame #4 {
                w1172 = ","
                n675 = local read "Computer Name"() -> (w1175:string)
                n676 = local read "Ver."() -> (w1174:string)
                n677 = property class="App"() -> ("App.Name"=w1171:string)  [unwired: 2 in, 2 out]
                n678 = local read "LAN IP Address"() -> (w1170:string)
                n679 = Concatenate Strings(w1170, w1172, w1175, w1172, w1171, w1172, w1174, w1172, "Stopped." ("string")) -> (w1169:string)
                n680 = call "Save Time to File.vi"("String"=w1169) -> ()  [unwired: 13 in, 2 out]
              }
              frame #5 {
                n681 = global read "Global HEWH.vi" "Test Station:"() -> (w1178:string)
                n682 = Concatenate Strings("robocopy c:/Data //10.2.0.10/AP2Lab/" ("command line"), w1178) -> (w1177:string)
                n683 = call <vilib>:"System Exec.vi"("run minimized? (F)"=TRUE, "command line"=w1177) -> ()  [unwired: 6 in, 4 out]
              }
            }
          }
        }
      }
      event "Help": Value Change {
        n684 = event-data() -> ()  [unwired: 1 in, 5 out]
        n685 = One Button Dialog(message="\n1.\tAfter unit has been stable for 30+/-5 minutes, Open valve, and draw 10.75 +/- .25 gallons of water at a rate of 3+/-.25 gpm.\n2.\tIf lower heat source energizes (Hybrid Mode/eHeat Mode = FAN ON follow by Compressor, Standard Electric Mode = Lower Element ON) before 10.75 gallons, then continue drawing water until Upper element engages as shown in step 5 (skip to step 5).\n3.\tIf lower heat source does not energize during 10.75 gallon draw, then wait a maximum of 10 minutes to see if lower heat source will energize.  If it does, then allow the water heater to recover to set point.\n4.\tAllow unit to sit 5 to 10 minutes in stabilized conditions, then:\n5.\tOpen valve and draw water at 3+/-.25 gpm until the Upper Element energizes.  Water draw must stop within 5 seconds after Upper Element energizes.  NOTE: when running the unit in e-Heat mode, (no upper element) draw 40+/-0.25 gallons of water.\n6.\tIn Hybrid Mode: when the Upper Element stops and switches to Lower Element, switch the unit to eHeat Mode.  This will switch the lower heating source to Compressor.\n7.\tAllow water heater to stabilize this second time. (Recover water temperature back to set point).\n8.\tAllow unit to sit a minimum of 30 minutes in stabilized conditions, then;\n9.\tStop Data Logger and HyperTerminal session. \n10.\tCapture all data into format shown in attached spreadsheet.\n\n\n") -> (true=w1184:bool)  [unwired: 1 in]
        n686 = Not(x=w1184) -> (.not. x?=w1183:bool)
        n687 = local write "Help"(w1183) -> ()
      }
    }
  }
